vi "Condition _string_4_prod_count_month.vi"(0 "From Date":timestamp format="%<%Y-%m-%d>T", 1 "Select Stakeholder":string(combo), 5 "To Date":timestamp format="%<%Y-%m-%d>T", 7 "Shift":string(combo)="ALL", 9 "Select Station":string(combo)="ST 1", 11 "STACKHOLDER_ID":i32, 12 "Refnum out 2":T1) -> (3 "Count":i32, 4 "sum":i32[](array[numeric]), 6 "ALL IN ONE":string[][](array[string]), 8 "Table":string[][](array[string]), 10 "Elements Found out":string[](array[string]), 13 "PROD_COUNT TEST":string[](array[string]), 14 "Refnum out":T1, 15 "Array 3":string[][](array[string]))   [LabVIEW 2017]
uses:
  <vilib>/addons/database/Connection.llb/Conn ObjectReference.ctl
  <vilib>/addons/database/NI_Database_API.lvlib
panel:
  in  "Array":string[](array[string])=["1", "2", "3", "4", "5", "6"]
  out "1":string[][](array[string])
  out "6":string[][](array[string])
  out "5":string[][](array[string])
  out "4":string[][](array[string])
  out "3":string[][](array[string])
  out "2":string[][](array[string])
  out "Array 2":string[][](array[string])
  in  "String":string="Select PLAN_DATE,PRODUCTION_COUNT,STATION_ID,DATE from "
  out "error out":errorcluster
  in  "error in (no error)":errorcluster
  # "2324"
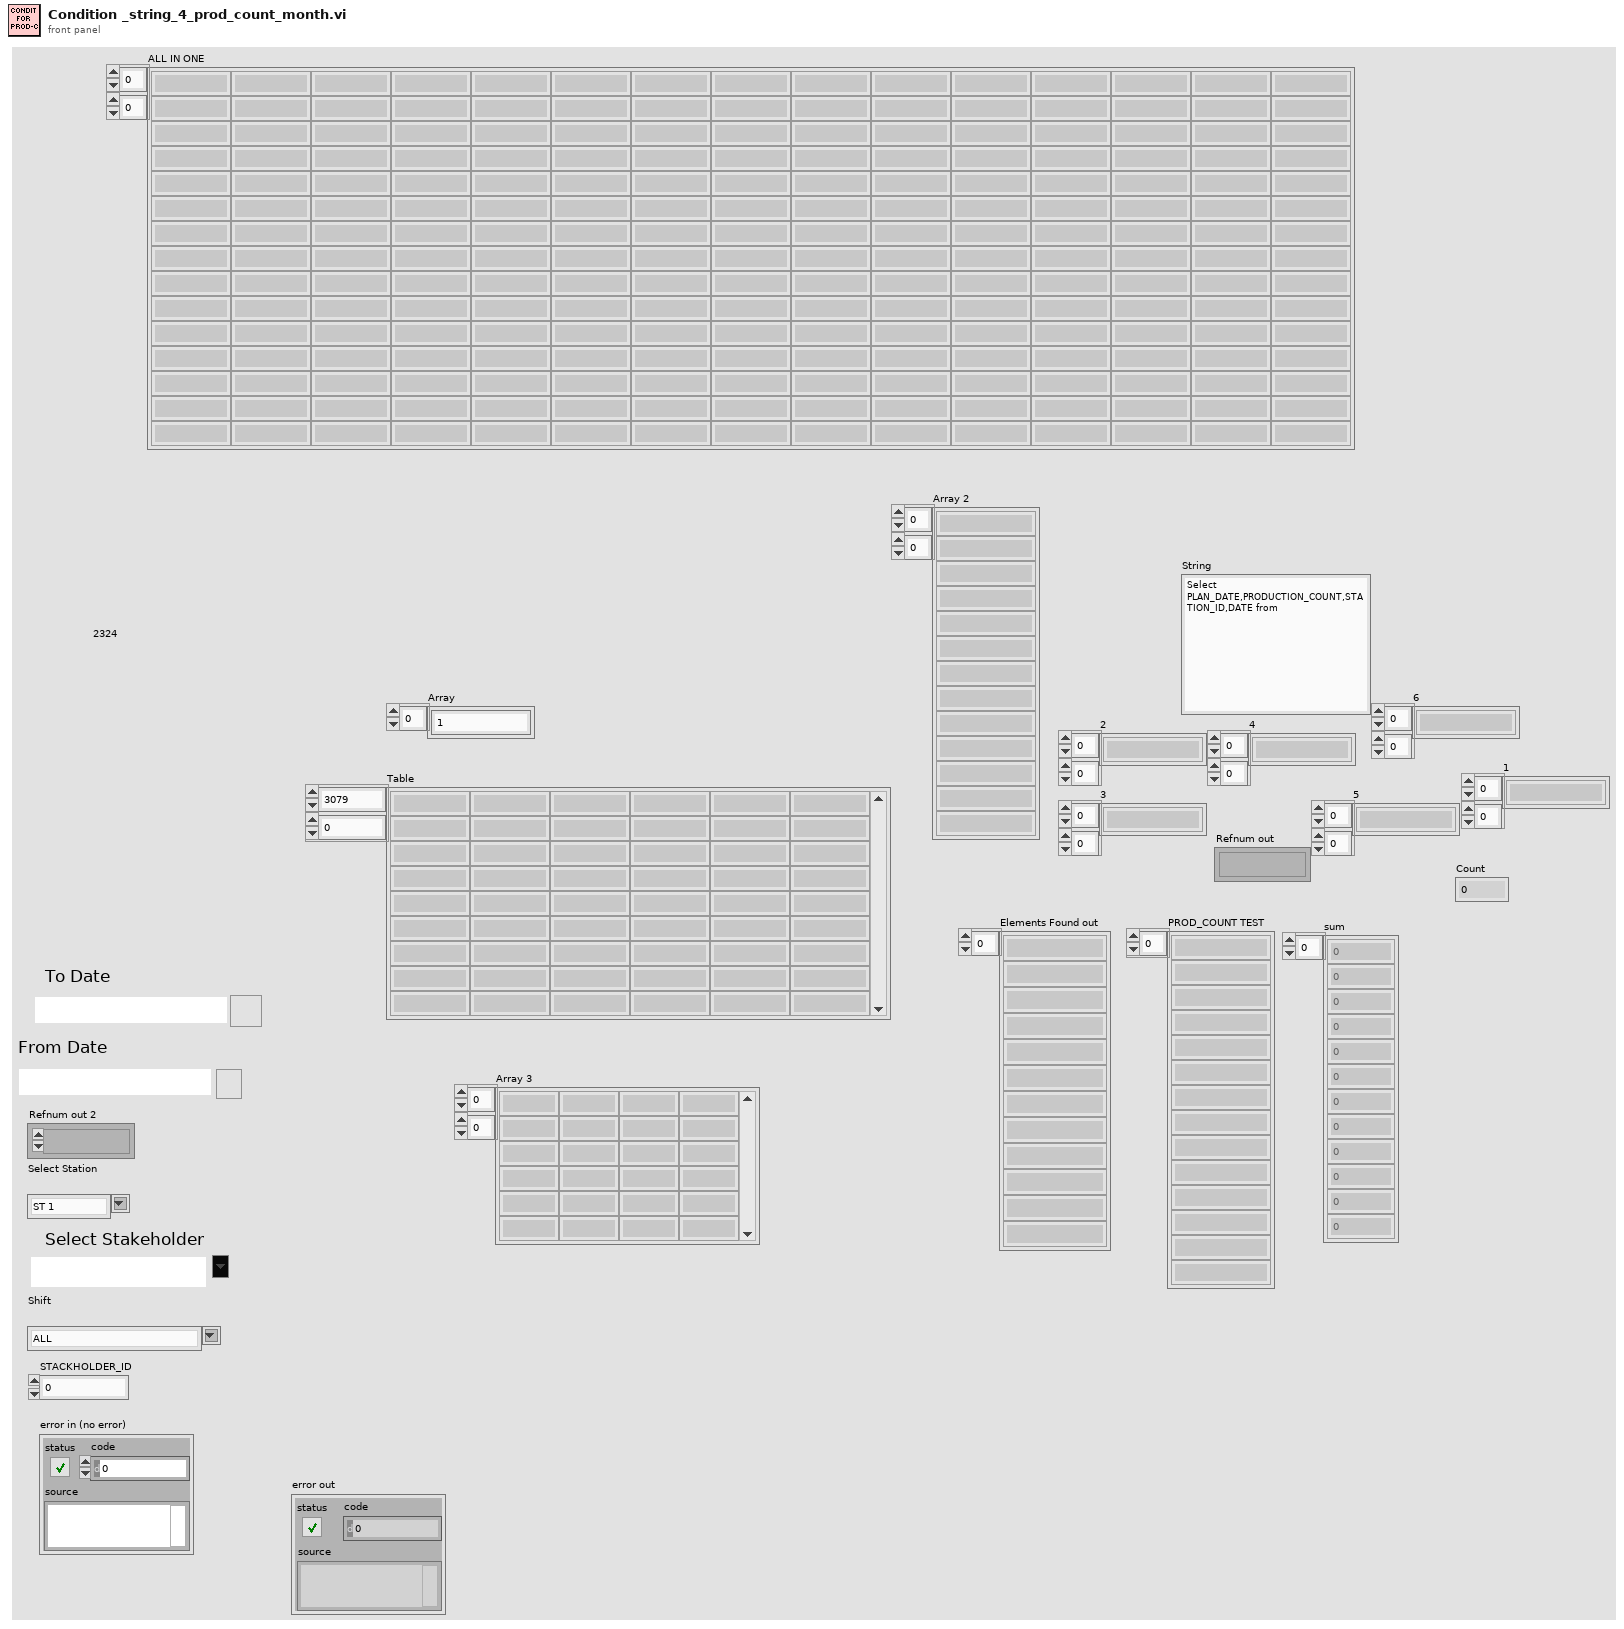
[diagram p1: front panel]
types:
  T1 = typedef "NI_Database_API.lvlib/Conn ObjectReference.ctl" = refnum<k1>
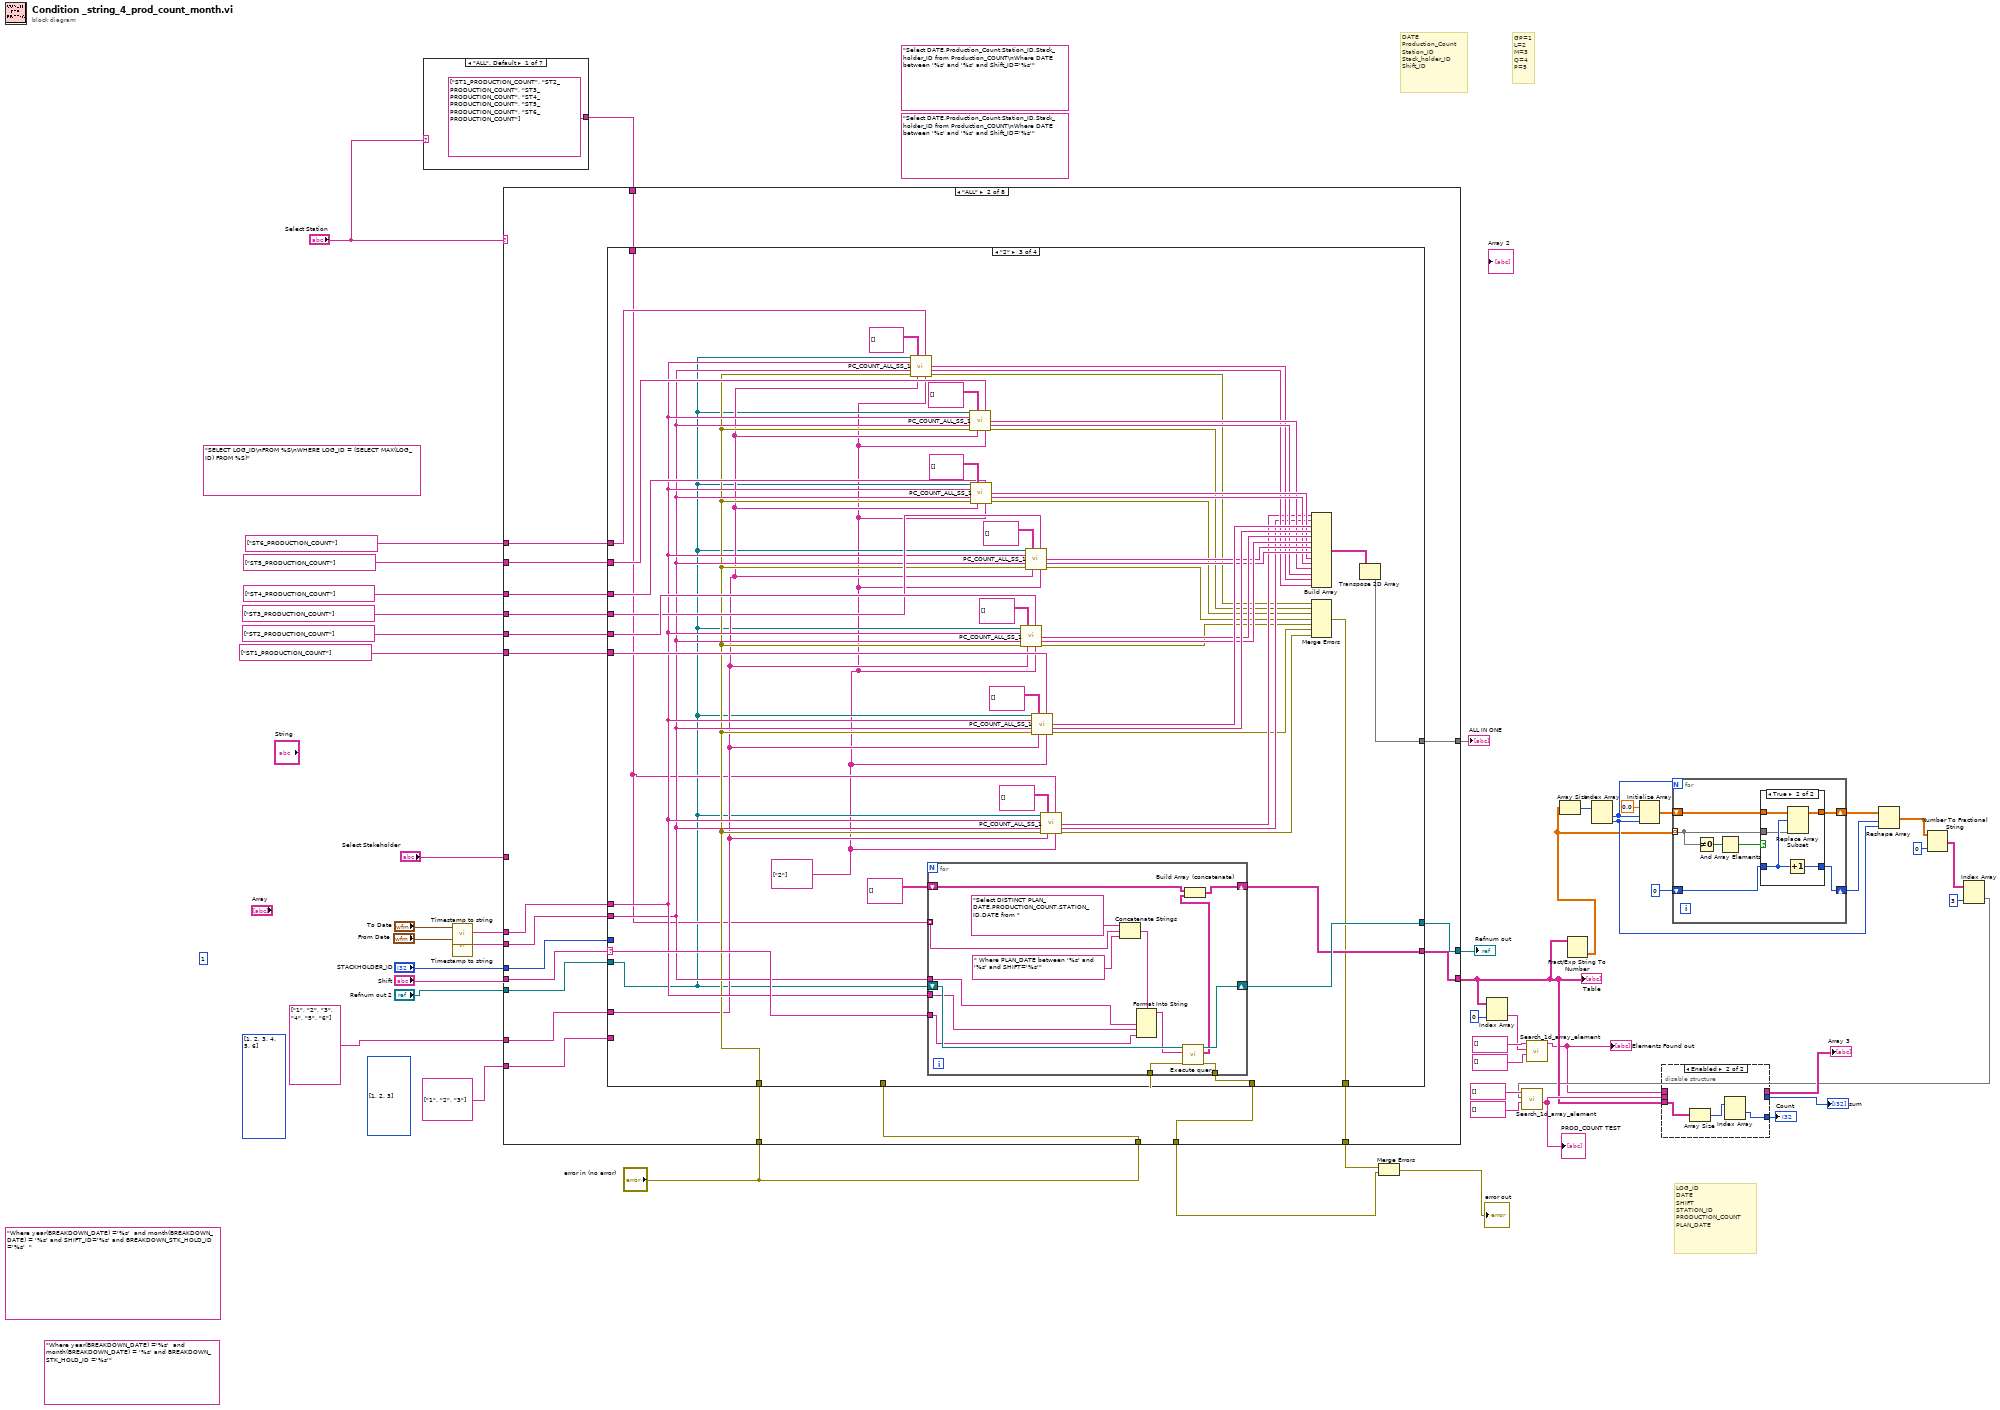
[diagram p0: block diagram]
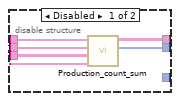
[diagram p2: hidden frame]
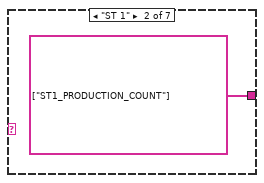
[diagram p4: hidden frame]
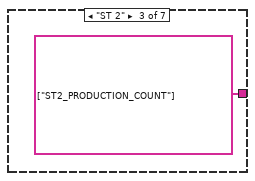
[diagram p5: hidden frame]
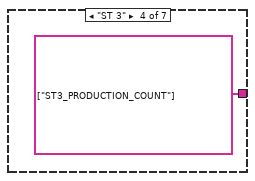
[diagram p6: hidden frame]
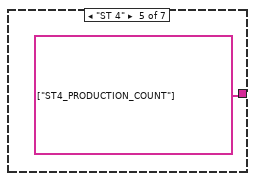
[diagram p7: hidden frame]
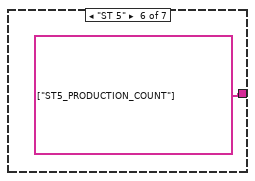
[diagram p8: hidden frame]
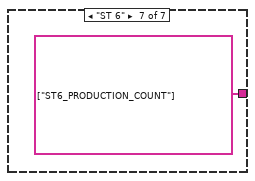
[diagram p9: hidden frame]
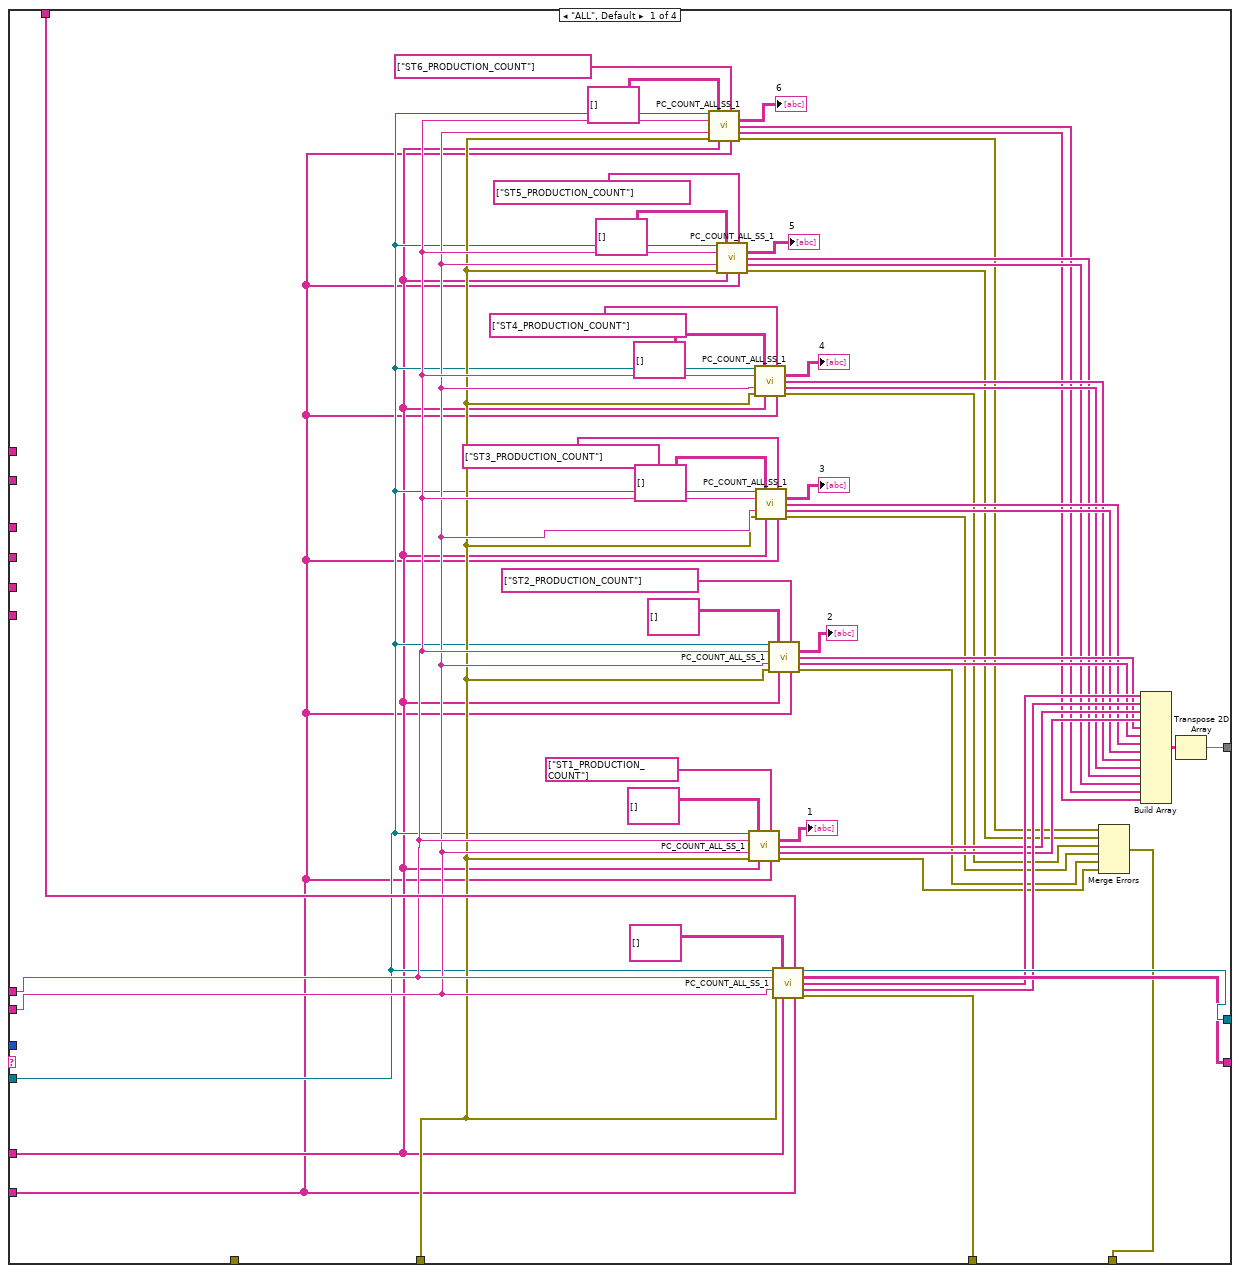
[diagram p11: hidden frame]
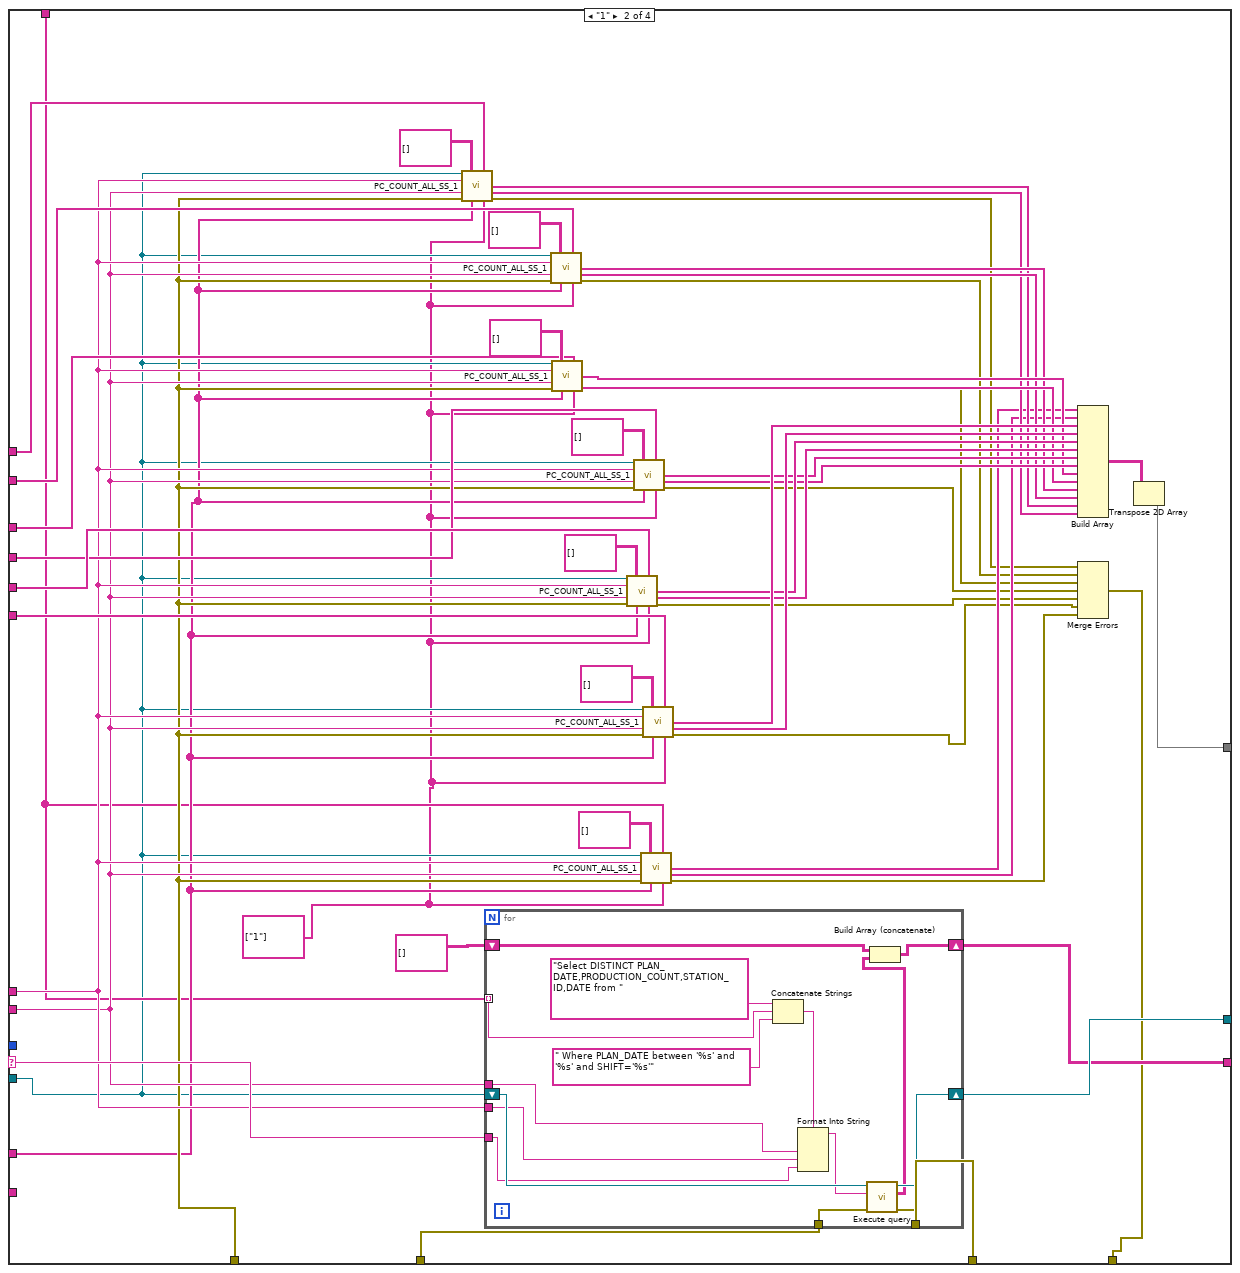
[diagram p12: hidden frame]
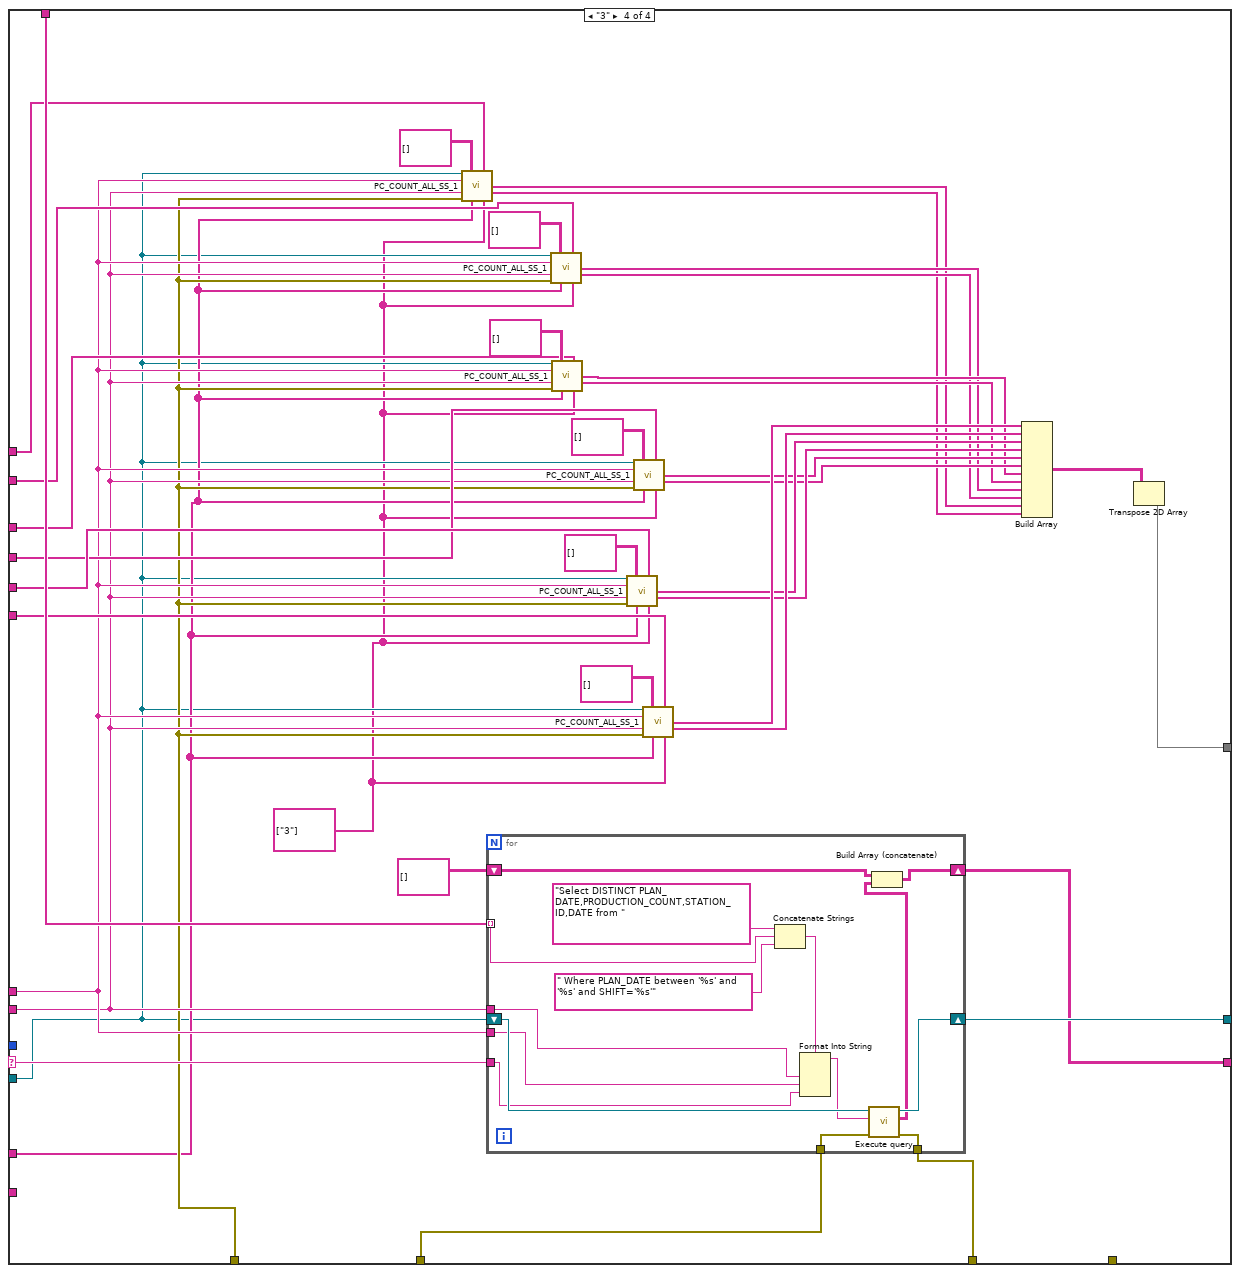
[diagram p13: hidden frame]
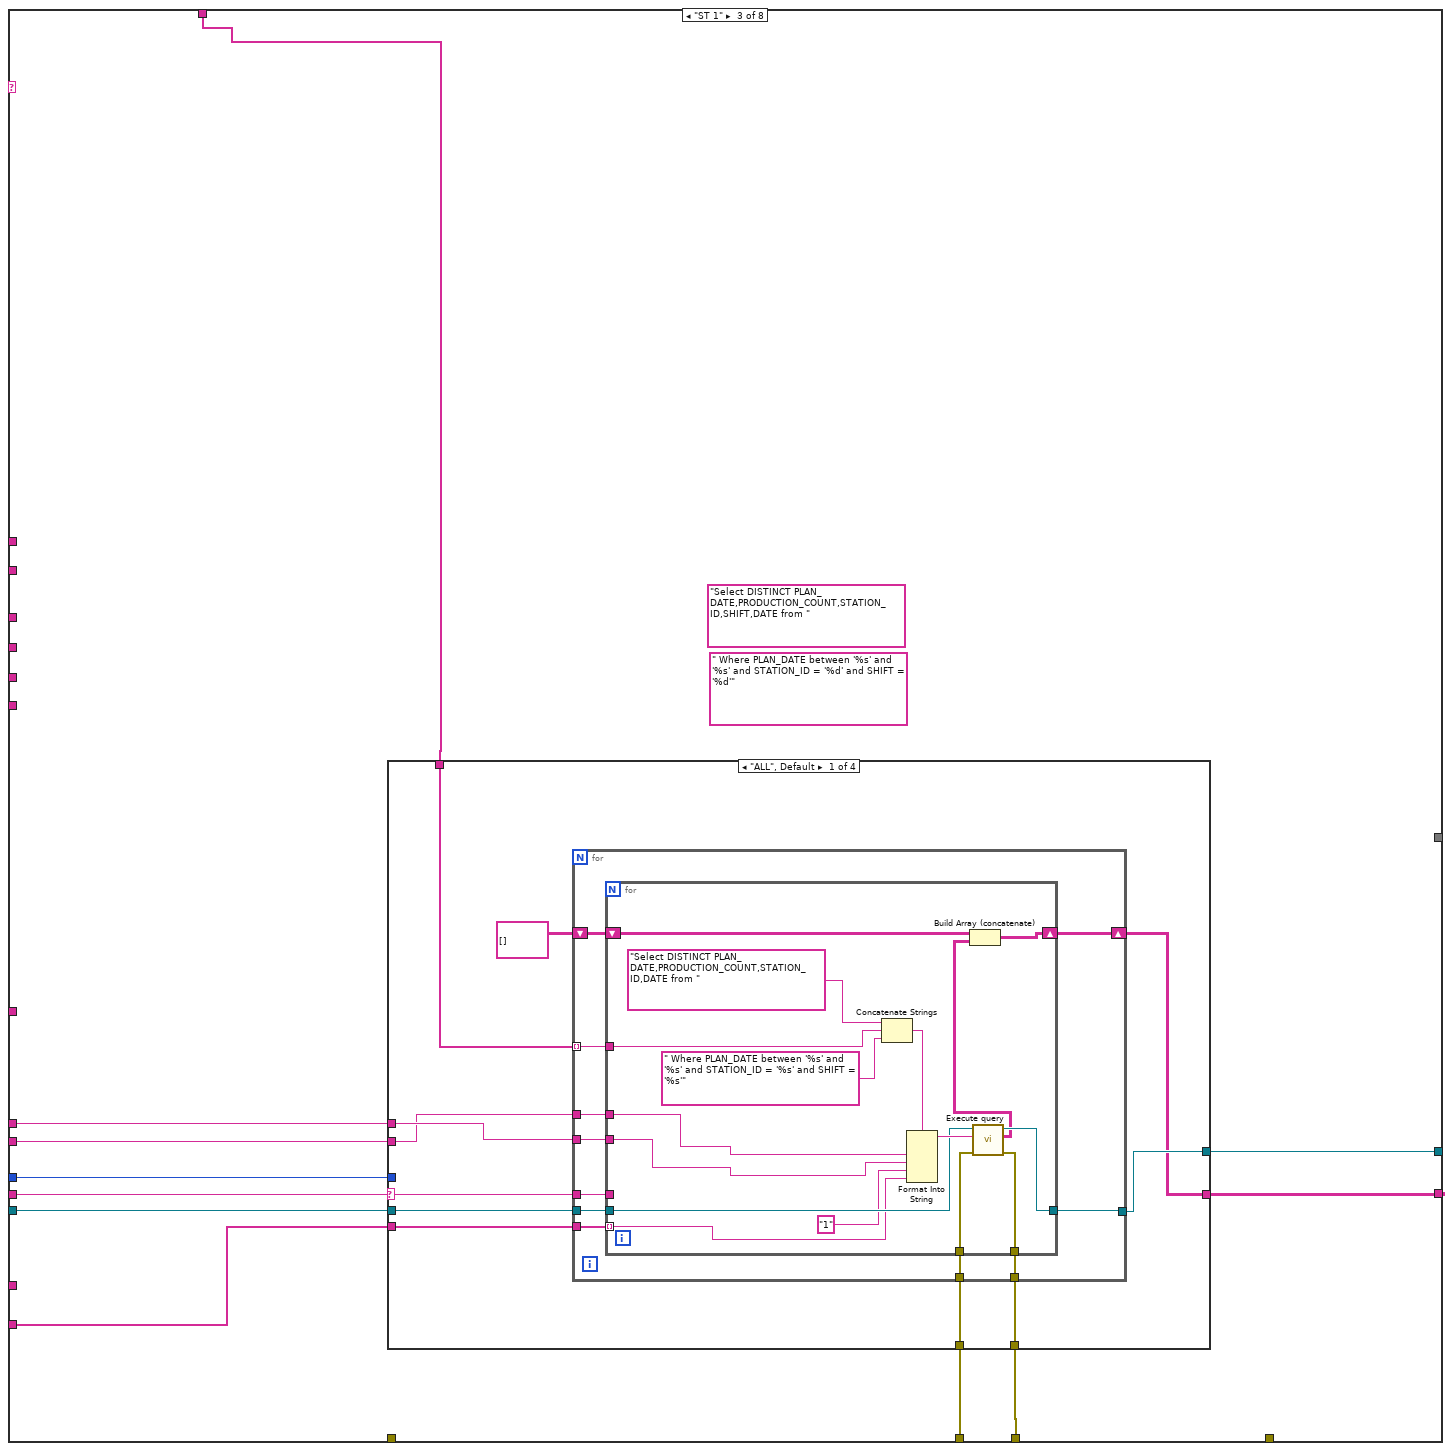
[diagram p14: hidden frame]
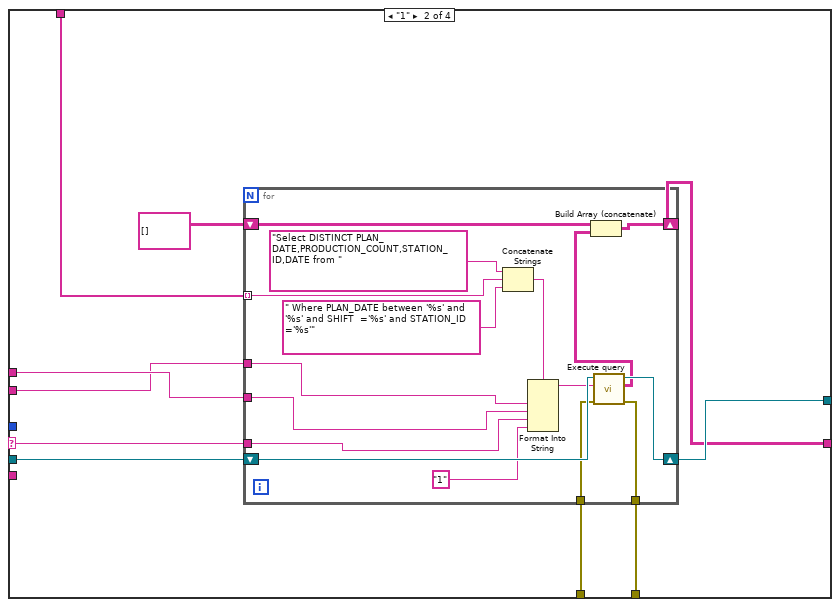
[diagram p15: hidden frame]
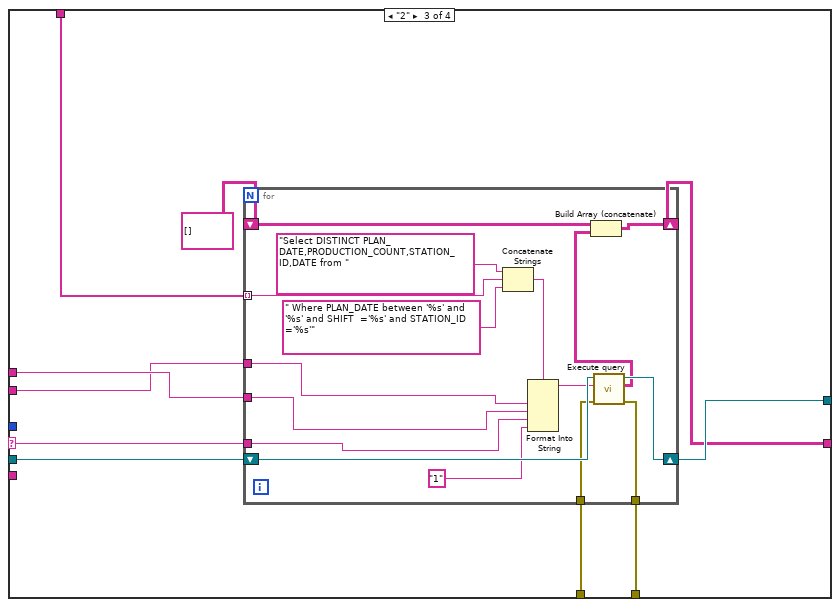
[diagram p16: hidden frame]
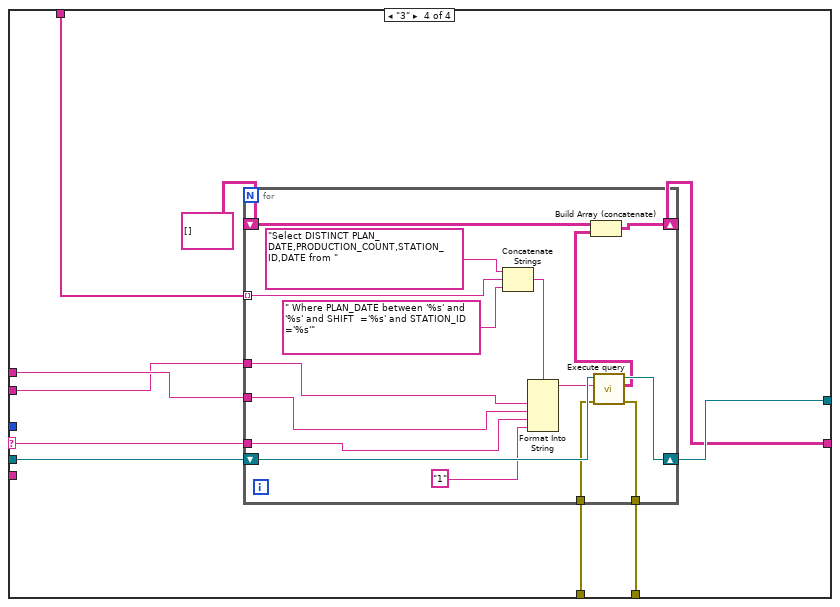
[diagram p17: hidden frame]
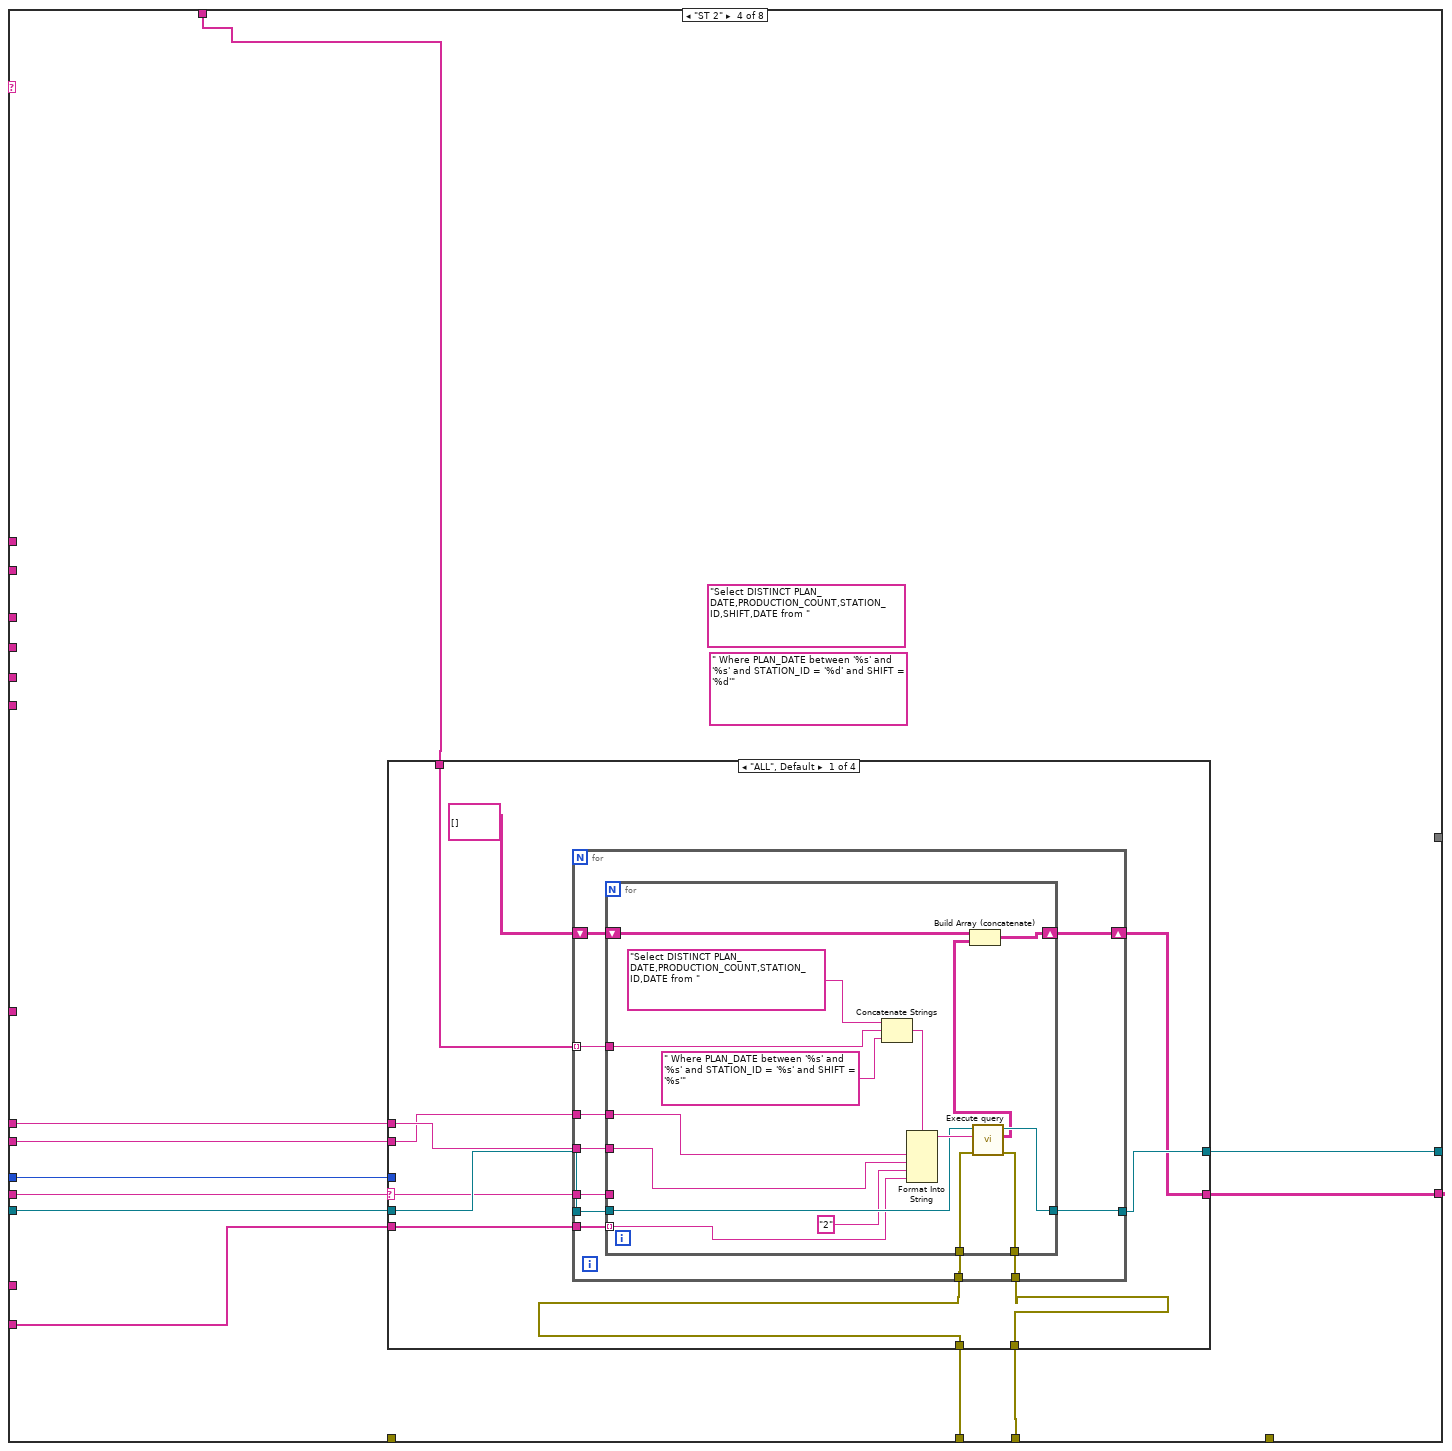
[diagram p18: hidden frame]
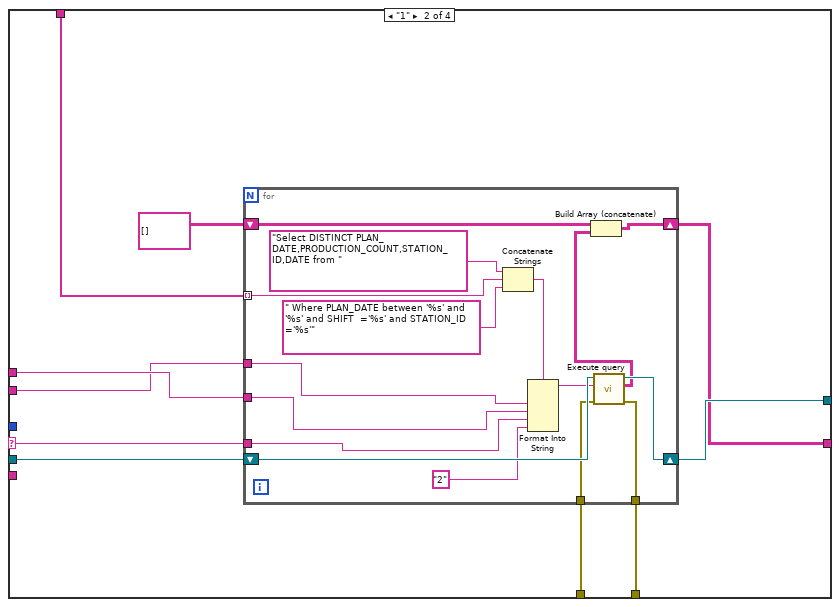
[diagram p19: hidden frame]
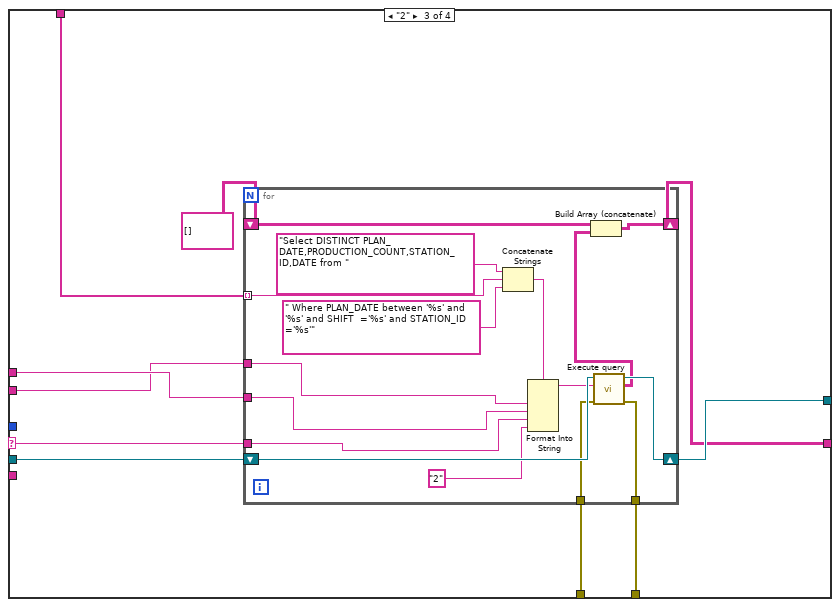
[diagram p20: hidden frame]
diagram:
  (unwired) 1
  (unwired) i32[] [1, 2, 3]
  (unwired) "SELECT LOG_ID\nFROM %S\nWHERE LOG_ID = (SELECT MAX(LOG_ID) FROM %S)" ("SQL query")
  (unwired) i32[] [1, 2, 3, 4, 5, 6]
  (unwired) "Select DATE,Production_Count,Station_ID,Stack_holder_ID from Production_COUNT\nWhere DATE between '%s' and '%s' and Shift_ID='%s'" ("string")
  (unwired) "Select DATE,Production_Count,Station_ID,Stack_holder_ID from Production_COUNT\nWhere DATE between '%s' and '%s' and Shift_ID='%s'" ("string")
  (unwired) "Where year(BREAKDOWN_DATE) ='%s'  and month(BREAKDOWN_DATE) = '%s' and BREAKDOWN_STK_HOLD_ID ='%s'" ("condition")
  (unwired) "Where year(BREAKDOWN_DATE) ='%s'  and month(BREAKDOWN_DATE) = '%s' and SHIFT_ID='%s' and BREAKDOWN_STK_HOLD_ID ='%s'  " ("condition")
  # "LOG_ID\nDATE\nSHIFT\nSTATION_ID\nPRODUCTION_COUNT\nPLAN_DATE"
  # "GP=1\nL=2\nM=3\nQ=4\nP=5"
  # "DATE\nProduction_Count\nStation_ID\nStack_holder_ID\nShift_ID"
  n1 = case shown="\"ALL\", Default" "Select Station" {
    tunnel: [string[] ["ST1_PRODUCTION_COUNT", "ST2_PRODUCTION_COUNT", "ST3_PRODUCTION_COUNT", "ST4_PRODUCTION_COUNT", "ST5_PRODUCTION_COUNT", "ST6_PRODUCTION_COUNT"] string[] ["ST1_PRODUCTION_COUNT"] string[] ["ST2_PRODUCTION_COUNT"] string[] ["ST3_PRODUCTION_COUNT"] string[] ["ST4_PRODUCTION_COUNT"] string[] ["ST5_PRODUCTION_COUNT"] string[] ["ST6_PRODUCTION_COUNT"]] -> w40
    frame "ALL", Default {
    }
    frame "ST 1" {
    }
    frame "ST 2" {
    }
    frame "ST 3" {
    }
    frame "ST 4" {
    }
    frame "ST 5" {
    }
    frame "ST 6" {
    }
  }
  n2 = call "Timestamp to string.vi"("time stamp"="To Date") -> ("Date"=w7:string)  [unwired: 8 in, 2 out]
  n3 = call "Timestamp to string.vi"("time stamp"="From Date") -> ("Date"=w5:string)  [unwired: 8 in, 2 out]
  n4 = case shown="\"ALL\"" "Select Station" {
    tunnel: "Shift" -> [_ w79 w326 w453 w580 w707 w834 w961]
    tunnel: w7 -> [_ w78 w325 w452 w579 w706 w833 w960]
    tunnel: w5 -> [_ w77 w324 w451 w578 w705 w832 w959]
    tunnel: "STACKHOLDER_ID" -> [_ w76 w323 w450 w577 w704 w831 w958]
    tunnel: [_ w75 w322 w449 w576 w703 w830 w957] -> w18
    tunnel: "Refnum out 2" -> [w58 w74 w321 w448 w575 w702 w829 w956]
    tunnel: [w58 w73 w320 w447 w574 w701 w828 w955] -> w47
    tunnel: "Select Stakeholder" -> [_ _ _ _ _ _ _ _]
    tunnel: w40 -> [_ w72 w319 w446 w573 w700 w827 w954]
    tunnel: "error in (no error)" -> [_ w71 w318 w445 w572 w699 w826 w953]
    tunnel: [_ w70 w317 w444 w571 w698 w825 w952] -> w28
    tunnel: string[] ["1", "2", "3", "4", "5", "6"] -> [_ w69 _ _ _ _ _ _]
    tunnel: string[] ["1", "2", "3"] -> [_ w68 w316 w443 w570 w697 w824 w951]
    tunnel: "error in (no error)" -> [_ w67 _ _ _ _ _ _]
    tunnel: [_ w66 _ _ _ _ _ _] -> w36
    tunnel: string[] ["ST1_PRODUCTION_COUNT"] ("Array 3") -> [_ w65 _ _ _ _ _ _]
    tunnel: string[] ["ST2_PRODUCTION_COUNT"] ("Array 3") -> [_ w64 _ _ _ _ _ _]
    tunnel: string[] ["ST3_PRODUCTION_COUNT"] ("Array 3") -> [_ w63 _ _ _ _ _ _]
    tunnel: string[] ["ST4_PRODUCTION_COUNT"] ("Array 3") -> [_ w62 _ _ _ _ _ _]
    tunnel: string[] ["ST5_PRODUCTION_COUNT"] ("Array 3") -> [_ w61 _ _ _ _ _ _]
    tunnel: string[] ["ST6_PRODUCTION_COUNT"] ("Array 3") -> [_ w60 _ _ _ _ _ _]
    tunnel: [_ w59 _ _ _ _ _ _] -> w29
    frame "False", Default {
    }
    frame "ALL" {
      n5 = case shown="\"2\"" w79 {
        selector: w79 -> [_ w180 w245 w299]
        tunnel: w78 -> [w110 w148 w213 w279]
        tunnel: w77 -> [w109 w147 w212 w278]
        tunnel: w76 -> [_ _ _ _]
        tunnel: [w127 w178 w243 w296] -> w75
        tunnel: w74 -> [w96 w141 w206 w275]
        tunnel: [w131 w181 w246 w300] -> w73
        tunnel: w72 -> [w130 w144 w209 w298]
        tunnel: w71 -> [w108 w177 w242 w295]
        tunnel: [w128 w176 w241 w294] -> w70
        tunnel: w69 -> [w94 w145 w210 w276]
        tunnel: w68 -> [w93 _ _ _]
        tunnel: w67 -> [_ w146 w211 w277]
        tunnel: [w95 w150 w215 w263] -> w66
        tunnel: w65 -> [_ w175 w240 w293]
        tunnel: w64 -> [_ w166 w231 w284]
        tunnel: w63 -> [_ w165 w230 w283]
        tunnel: w62 -> [_ w164 w229 w282]
        tunnel: w61 -> [_ w163 w228 w281]
        tunnel: w60 -> [_ w162 w227 w280]
        tunnel: [w86 w133 w198 _] -> w59
        frame "ALL", Default {
          n6 = call "PC_COUNT_ALL_SS_1.vi"("Refnum in"=w96, "data in"=string[][] [] ("data"), "Array 3"=string[] ["ST6_PRODUCTION_COUNT"], "To Date"=w110, "From Date"=w109, "error in (no error)"=w108, "Station"=w94, "Shift"=w93) -> ("data out"=→"6":string[][], "DATE"=w99:string[], "COUNT"=w98:string[], "error out"=w92:errorcluster)  [unwired: 3 in, 1 out]
          n7 = call "PC_COUNT_ALL_SS_1.vi"("Refnum in"=w96, "data in"=string[][] [] ("data"), "Array 3"=string[] ["ST5_PRODUCTION_COUNT"], "To Date"=w110, "From Date"=w109, "error in (no error)"=w108, "Station"=w94, "Shift"=w93) -> ("data out"=→"5":string[][], "DATE"=w101:string[], "COUNT"=w100:string[], "error out"=w91:errorcluster)  [unwired: 3 in, 1 out]
          n8 = call "PC_COUNT_ALL_SS_1.vi"("Refnum in"=w96, "data in"=string[][] [] ("data"), "Array 3"=string[] ["ST1_PRODUCTION_COUNT"], "To Date"=w110, "From Date"=w109, "error in (no error)"=w108, "Station"=w94, "Shift"=w93) -> ("data out"=→"1":string[][], "DATE"=w122:string[], "COUNT"=w121:string[], "error out"=w87:errorcluster)  [unwired: 3 in, 1 out]
          n9 = call "PC_COUNT_ALL_SS_1.vi"("Refnum in"=w96, "data in"=string[][] [] ("data"), "Array 3"=string[] ["ST4_PRODUCTION_COUNT"], "To Date"=w110, "From Date"=w109, "error in (no error)"=w108, "Station"=w94, "Shift"=w93) -> ("data out"=→"4":string[][], "DATE"=w103:string[], "COUNT"=w102:string[], "error out"=w90:errorcluster)  [unwired: 3 in, 1 out]
          n10 = call "PC_COUNT_ALL_SS_1.vi"("Refnum in"=w96, "data in"=string[][] [] ("data"), "Array 3"=string[] ["ST3_PRODUCTION_COUNT"], "To Date"=w110, "From Date"=w109, "error in (no error)"=w108, "Station"=w94, "Shift"=w93) -> ("data out"=→"3":string[][], "DATE"=w105:string[], "COUNT"=w104:string[], "error out"=w89:errorcluster)  [unwired: 3 in, 1 out]
          n11 = call "PC_COUNT_ALL_SS_1.vi"("Refnum in"=w96, "data in"=string[][] [] ("data"), "Array 3"=string[] ["ST2_PRODUCTION_COUNT"], "To Date"=w110, "From Date"=w109, "error in (no error)"=w108, "Station"=w94, "Shift"=w93) -> ("data out"=→"2":string[][], "DATE"=w118:string[], "COUNT"=w117:string[], "error out"=w88:errorcluster)  [unwired: 3 in, 1 out]
          n12 = call "PC_COUNT_ALL_SS_1.vi"("Refnum in"=w96, "data in"=string[][] [] ("data"), "Array 3"=w130, "To Date"=w110, "From Date"=w109, "error in (no error)"=w108, "Station"=w94, "Shift"=w93) -> ("Refnum out"=w131:T1, "data out"=w127:string[][], "DATE"=w124:string[], "COUNT"=w123:string[], "error out"=w128:errorcluster)  [unwired: 3 in]
          n13 = Merge Errors(w92, w91, w90, w89, w88, w87) -> (w86:errorcluster)
          n14 = Build Array(w124, w123, w122, w121, w118, w117, w105, w104, w103, w102, w101, w100, w99, w98) -> (w97:string[][])
          n15 = Transpose 2D Array(2D array=w97) -> (transposed array=w95:string[][])
        }
        frame "1" {
          w132 = string[] ["1"]
          n16 = call "PC_COUNT_ALL_SS_1.vi"("Refnum in"=w141, "data in"=string[][] [], "Array 3"=w162, "To Date"=w148, "From Date"=w147, "error in (no error)"=w146, "Station"=w145, "Shift"=w132) -> ("DATE"=w153:string[], "COUNT"=w152:string[], "error out"=w140:errorcluster)  [unwired: 3 in, 2 out]
          n17 = for {
            tunnel: w148 -> [w182]
            tunnel: w147 -> [w183]
            tunnel: w180 -> [w193]
            shift-right: [w194] -> w181
            shift-left: w141 -> [w196]
            tunnel: w144 -> [w191] mode=indexing
            shift-right: [w187] -> w178
            shift-left: string[][] [] ("data") -> [w188]
            tunnel: w177 -> [w185]
            tunnel: [w184] -> w176
            n18 = Concatenate Strings("Select DISTINCT PLAN_DATE,PRODUCTION_COUNT,STATION_ID,DATE from ", w191, " Where PLAN_DATE between '%s' and '%s' and SHIFT='%s'") -> (w192:string)
            n19 = Format Into String(format string=w192, w183, w182, w193) -> (resulting string=w195:string)  [unwired: 2 in, 1 out]
            n20 = call "Execute query.vi"("error in (no error)"=w185, "String"=w195, "connection reference"=w196) -> ("error out"=w184:errorcluster, "Table"=w186:string[][], "connection reference 2"=w194:T1)  [unwired: 3 in, 3 out]
            n21 = Build Array (concatenate)(w188, w186) -> (w187:string[][])
          }
          n22 = call "PC_COUNT_ALL_SS_1.vi"("Refnum in"=w141, "data in"=string[][] [], "Array 3"=w163, "To Date"=w148, "From Date"=w147, "error in (no error)"=w146, "Station"=w145, "Shift"=w132) -> ("DATE"=w155:string[], "COUNT"=w154:string[], "error out"=w139:errorcluster)  [unwired: 3 in, 2 out]
          n23 = call "PC_COUNT_ALL_SS_1.vi"("Refnum in"=w141, "data in"=string[][] [], "Array 3"=w164, "To Date"=w148, "From Date"=w147, "error in (no error)"=w146, "Station"=w145, "Shift"=w132) -> ("DATE"=w157:string[], "COUNT"=w156:string[], "error out"=w138:errorcluster)  [unwired: 3 in, 2 out]
          n24 = call "PC_COUNT_ALL_SS_1.vi"("Refnum in"=w141, "data in"=string[][] [], "Array 3"=w166, "To Date"=w148, "From Date"=w147, "error in (no error)"=w146, "Station"=w145, "Shift"=w132) -> ("DATE"=w161:string[], "COUNT"=w160:string[], "error out"=w136:errorcluster)  [unwired: 3 in, 2 out]
          n25 = call "PC_COUNT_ALL_SS_1.vi"("Refnum in"=w141, "data in"=string[][] [], "Array 3"=w165, "To Date"=w148, "From Date"=w147, "error in (no error)"=w146, "Station"=w145, "Shift"=w132) -> ("DATE"=w159:string[], "COUNT"=w158:string[], "error out"=w137:errorcluster)  [unwired: 3 in, 2 out]
          n26 = call "PC_COUNT_ALL_SS_1.vi"("Refnum in"=w141, "data in"=string[][] [], "Array 3"=w144, "To Date"=w148, "From Date"=w147, "error in (no error)"=w146, "Station"=w145, "Shift"=w132) -> ("DATE"=w143:string[], "COUNT"=w142:string[], "error out"=w134:errorcluster)  [unwired: 3 in, 2 out]
          n27 = call "PC_COUNT_ALL_SS_1.vi"("Refnum in"=w141, "data in"=string[][] [], "Array 3"=w175, "To Date"=w148, "From Date"=w147, "error in (no error)"=w146, "Station"=w145, "Shift"=w132) -> ("DATE"=w173:string[], "COUNT"=w172:string[], "error out"=w135:errorcluster)  [unwired: 3 in, 2 out]
          n28 = Build Array(w143, w142, w173, w172, w161, w160, w159, w158, w157, w156, w155, w154, w153, w152) -> (w151:string[][])
          n29 = Merge Errors(w140, w139, w138, w137, w136, w135, w134) -> (w133:errorcluster)
          n30 = Transpose 2D Array(2D array=w151) -> (transposed array=w150:string[][])
        }
        frame "2" {
          w197 = string[] ["2"]
          n31 = call "PC_COUNT_ALL_SS_1.vi"("Refnum in"=w206, "data in"=string[][] [], "Array 3"=w227, "To Date"=w213, "From Date"=w212, "error in (no error)"=w211, "Station"=w210, "Shift"=w197) -> ("DATE"=w218:string[], "COUNT"=w217:string[], "error out"=w205:errorcluster)  [unwired: 3 in, 2 out]
          n32 = for {
            tunnel: w213 -> [w247]
            tunnel: w212 -> [w248]
            tunnel: w245 -> [w258]
            shift-right: [w259] -> w246
            shift-left: w206 -> [w261]
            tunnel: w209 -> [w256] mode=indexing
            shift-right: [w252] -> w243
            shift-left: string[][] [] ("data") -> [w253]
            tunnel: w242 -> [w250]
            tunnel: [w249] -> w241
            n33 = Concatenate Strings("Select DISTINCT PLAN_DATE,PRODUCTION_COUNT,STATION_ID,DATE from ", w256, " Where PLAN_DATE between '%s' and '%s' and SHIFT='%s'") -> (w257:string)
            n34 = Format Into String(format string=w257, w248, w247, w258) -> (resulting string=w260:string)  [unwired: 2 in, 1 out]
            n35 = call "Execute query.vi"("error in (no error)"=w250, "String"=w260, "connection reference"=w261) -> ("error out"=w249:errorcluster, "Table"=w251:string[][], "connection reference 2"=w259:T1)  [unwired: 3 in, 3 out]
            n36 = Build Array (concatenate)(w253, w251) -> (w252:string[][])
          }
          n37 = call "PC_COUNT_ALL_SS_1.vi"("Refnum in"=w206, "data in"=string[][] [], "Array 3"=w228, "To Date"=w213, "From Date"=w212, "error in (no error)"=w211, "Station"=w210, "Shift"=w197) -> ("DATE"=w220:string[], "COUNT"=w219:string[], "error out"=w204:errorcluster)  [unwired: 3 in, 2 out]
          n38 = call "PC_COUNT_ALL_SS_1.vi"("Refnum in"=w206, "data in"=string[][] [], "Array 3"=w229, "To Date"=w213, "From Date"=w212, "error in (no error)"=w211, "Station"=w210, "Shift"=w197) -> ("DATE"=w222:string[], "COUNT"=w221:string[], "error out"=w203:errorcluster)  [unwired: 3 in, 2 out]
          n39 = call "PC_COUNT_ALL_SS_1.vi"("Refnum in"=w206, "data in"=string[][] [], "Array 3"=w231, "To Date"=w213, "From Date"=w212, "error in (no error)"=w211, "Station"=w210, "Shift"=w197) -> ("DATE"=w226:string[], "COUNT"=w225:string[], "error out"=w201:errorcluster)  [unwired: 3 in, 2 out]
          n40 = call "PC_COUNT_ALL_SS_1.vi"("Refnum in"=w206, "data in"=string[][] [], "Array 3"=w230, "To Date"=w213, "From Date"=w212, "error in (no error)"=w211, "Station"=w210, "Shift"=w197) -> ("DATE"=w224:string[], "COUNT"=w223:string[], "error out"=w202:errorcluster)  [unwired: 3 in, 2 out]
          n41 = call "PC_COUNT_ALL_SS_1.vi"("Refnum in"=w206, "data in"=string[][] [], "Array 3"=w240, "To Date"=w213, "From Date"=w212, "error in (no error)"=w211, "Station"=w210, "Shift"=w197) -> ("DATE"=w238:string[], "COUNT"=w237:string[], "error out"=w200:errorcluster)  [unwired: 3 in, 2 out]
          n42 = call "PC_COUNT_ALL_SS_1.vi"("Refnum in"=w206, "data in"=string[][] [], "Array 3"=w209, "To Date"=w213, "From Date"=w212, "error in (no error)"=w211, "Station"=w210, "Shift"=w197) -> ("DATE"=w208:string[], "COUNT"=w207:string[], "error out"=w199:errorcluster)  [unwired: 3 in, 2 out]
          n43 = Build Array(w208, w207, w238, w237, w226, w225, w224, w223, w222, w221, w220, w219, w218, w217) -> (w216:string[][])
          n44 = Merge Errors(w205, w204, w203, w202, w201, w200, w199) -> (w198:errorcluster)
          n45 = Transpose 2D Array(2D array=w216) -> (transposed array=w215:string[][])
        }
        frame "3" {
          w262 = string[] ["3"]
          n46 = call "PC_COUNT_ALL_SS_1.vi"("Refnum in"=w275, "data in"=string[][] [], "Array 3"=w280, "To Date"=w279, "From Date"=w278, "error in (no error)"=w277, "Station"=w276, "Shift"=w262) -> ("DATE"=w266:string[], "COUNT"=w265:string[])  [unwired: 3 in, 3 out]
          n47 = for {
            tunnel: w279 -> [w301]
            tunnel: w278 -> [w302]
            tunnel: w299 -> [w312]
            shift-right: [w313] -> w300
            shift-left: w275 -> [w315]
            tunnel: w298 -> [w310] mode=indexing
            shift-right: [w306] -> w296
            shift-left: string[][] [] ("data") -> [w307]
            tunnel: w295 -> [w304]
            tunnel: [w303] -> w294
            n48 = Concatenate Strings("Select DISTINCT PLAN_DATE,PRODUCTION_COUNT,STATION_ID,DATE from ", w310, " Where PLAN_DATE between '%s' and '%s' and SHIFT='%s'") -> (w311:string)
            n49 = Format Into String(format string=w311, w302, w301, w312) -> (resulting string=w314:string)  [unwired: 2 in, 1 out]
            n50 = call "Execute query.vi"("error in (no error)"=w304, "String"=w314, "connection reference"=w315) -> ("error out"=w303:errorcluster, "Table"=w305:string[][], "connection reference 2"=w313:T1)  [unwired: 3 in, 3 out]
            n51 = Build Array (concatenate)(w307, w305) -> (w306:string[][])
          }
          n52 = call "PC_COUNT_ALL_SS_1.vi"("Refnum in"=w275, "data in"=string[][] [], "Array 3"=w281, "To Date"=w279, "From Date"=w278, "error in (no error)"=w277, "Station"=w276, "Shift"=w262) -> ("DATE"=w268:string[], "COUNT"=w267:string[])  [unwired: 3 in, 3 out]
          n53 = call "PC_COUNT_ALL_SS_1.vi"("Refnum in"=w275, "data in"=string[][] [], "Array 3"=w282, "To Date"=w279, "From Date"=w278, "error in (no error)"=w277, "Station"=w276, "Shift"=w262) -> ("DATE"=w270:string[], "COUNT"=w269:string[])  [unwired: 3 in, 3 out]
          n54 = call "PC_COUNT_ALL_SS_1.vi"("Refnum in"=w275, "data in"=string[][] [], "Array 3"=w284, "To Date"=w279, "From Date"=w278, "error in (no error)"=w277, "Station"=w276, "Shift"=w262) -> ("DATE"=w274:string[], "COUNT"=w273:string[])  [unwired: 3 in, 3 out]
          n55 = call "PC_COUNT_ALL_SS_1.vi"("Refnum in"=w275, "data in"=string[][] [], "Array 3"=w283, "To Date"=w279, "From Date"=w278, "error in (no error)"=w277, "Station"=w276, "Shift"=w262) -> ("DATE"=w272:string[], "COUNT"=w271:string[])  [unwired: 3 in, 3 out]
          n56 = call "PC_COUNT_ALL_SS_1.vi"("Refnum in"=w275, "data in"=string[][] [], "Array 3"=w293, "To Date"=w279, "From Date"=w278, "error in (no error)"=w277, "Station"=w276, "Shift"=w262) -> ("DATE"=w291:string[], "COUNT"=w290:string[])  [unwired: 3 in, 3 out]
          n57 = Build Array(w291, w290, w274, w273, w272, w271, w270, w269, w268, w267, w266, w265) -> (w264:string[][])
          n58 = Transpose 2D Array(2D array=w264) -> (transposed array=w263:string[][])
        }
      }
    }
    frame "ST 1" {
      (unwired) "Select DISTINCT PLAN_DATE,PRODUCTION_COUNT,STATION_ID,SHIFT,DATE from "
      (unwired) " Where PLAN_DATE between '%s' and '%s' and STATION_ID = '%d' and SHIFT = '%d'"
      n59 = case shown="\"ALL\", Default" w326 {
        selector: w326 -> [w333 w370 w396 w422]
        tunnel: w325 -> [w337 w374 w400 w426]
        tunnel: w324 -> [w336 w373 w399 w425]
        tunnel: w323 -> [_ _ _ _]
        tunnel: [w328 w367 w393 w419] -> w322
        tunnel: w321 -> [w335 w372 w398 w424]
        tunnel: [w334 w371 w397 w423] -> w320
        tunnel: w319 -> [w332 w369 w395 w421]
        tunnel: w318 -> [w330 w365 w392 w418]
        tunnel: [w329 w366 w391 w417] -> w317
        tunnel: w316 -> [w327 _ _ _]
        frame "ALL", Default {
          n60 = for {
            tunnel: w337 -> [w348]
            tunnel: w336 -> [w347]
            tunnel: w333 -> [w344]
            tunnel: w332 -> [w343] mode=indexing
            tunnel: w330 -> [w341]
            tunnel: [w340] -> w329
            tunnel: w335 -> [w346]
            tunnel: [w345] -> w334
            shift-right: [w339] -> w328
            shift-left: string[][] [] ("data") -> [w342]
            tunnel: w327 -> [w338]
            n61 = for {
              tunnel: w348 -> [w349]
              tunnel: w347 -> [w350]
              tunnel: w344 -> [_]
              tunnel: w343 -> [w362]
              shift-right: [w352] -> w339
              shift-left: w342 -> [w359]
              tunnel: w341 -> [w355]
              tunnel: [w354] -> w340
              tunnel: w346 -> [w357]
              tunnel: [w363] -> w345
              tunnel: w338 -> [w351] mode=indexing
              n62 = Concatenate Strings("Select DISTINCT PLAN_DATE,PRODUCTION_COUNT,STATION_ID,DATE from ", w362, " Where PLAN_DATE between '%s' and '%s' and STATION_ID = '%s' and SHIFT = '%s'") -> (w360:string)
              n63 = Format Into String(format string=w360, w350, w349, "1", w351) -> (resulting string=w364:string)  [unwired: 2 in, 1 out]
              n64 = call "Execute query.vi"("error in (no error)"=w355, "String"=w364, "connection reference"=w357) -> ("error out"=w354:errorcluster, "Table"=w358:string[][], "connection reference 2"=w363:T1)  [unwired: 3 in, 3 out]
              n65 = Build Array (concatenate)(w359, w358) -> (w352:string[][])
            }
          }
        }
        frame "1" {
          n66 = for {
            tunnel: w374 -> [w375]
            tunnel: w373 -> [w376]
            tunnel: w370 -> [w387]
            tunnel: w369 -> [w386] mode=indexing
            shift-right: [w388] -> w371
            shift-left: w372 -> [w390]
            shift-right: [w381] -> w367
            shift-left: string[][] [] ("data") -> [w383]
            tunnel: [w378] -> w366
            tunnel: w365 -> [w377]
            n67 = Concatenate Strings("Select DISTINCT PLAN_DATE,PRODUCTION_COUNT,STATION_ID,DATE from ", w386, " Where PLAN_DATE between '%s' and '%s' and SHIFT  ='%s' and STATION_ID ='%s'") -> (w384:string)
            n68 = Format Into String(format string=w384, w376, w375, w387, "1") -> (resulting string=w389:string)  [unwired: 2 in, 1 out]
            n69 = call "Execute query.vi"("error in (no error)"=w377, "String"=w389, "connection reference"=w390) -> ("error out"=w378:errorcluster, "Table"=w382:string[][], "connection reference 2"=w388:T1)  [unwired: 3 in, 3 out]
            n70 = Build Array (concatenate)(w383, w382) -> (w381:string[][])
          }
        }
        frame "2" {
          n71 = for {
            tunnel: w400 -> [w401]
            tunnel: w399 -> [w402]
            tunnel: w396 -> [w413]
            tunnel: w395 -> [w412] mode=indexing
            shift-right: [w414] -> w397
            shift-left: w398 -> [w416]
            shift-right: [w407] -> w393
            shift-left: string[][] [] ("data") -> [w409]
            tunnel: w392 -> [w404]
            tunnel: [w403] -> w391
            n72 = Concatenate Strings("Select DISTINCT PLAN_DATE,PRODUCTION_COUNT,STATION_ID,DATE from ", w412, " Where PLAN_DATE between '%s' and '%s' and SHIFT  ='%s' and STATION_ID ='%s'") -> (w410:string)
            n73 = Format Into String(format string=w410, w402, w401, w413, "1") -> (resulting string=w415:string)  [unwired: 2 in, 1 out]
            n74 = call "Execute query.vi"("error in (no error)"=w404, "String"=w415, "connection reference"=w416) -> ("error out"=w403:errorcluster, "Table"=w408:string[][], "connection reference 2"=w414:T1)  [unwired: 3 in, 3 out]
            n75 = Build Array (concatenate)(w409, w408) -> (w407:string[][])
          }
        }
        frame "3" {
          n76 = for {
            tunnel: w426 -> [w427]
            tunnel: w425 -> [w428]
            tunnel: w422 -> [w439]
            tunnel: w421 -> [w438] mode=indexing
            shift-right: [w440] -> w423
            shift-left: w424 -> [w442]
            shift-right: [w433] -> w419
            shift-left: string[][] [] ("data") -> [w435]
            tunnel: w418 -> [w430]
            tunnel: [w429] -> w417
            n77 = Concatenate Strings("Select DISTINCT PLAN_DATE,PRODUCTION_COUNT,STATION_ID,DATE from ", w438, " Where PLAN_DATE between '%s' and '%s' and SHIFT  ='%s' and STATION_ID ='%s'") -> (w436:string)
            n78 = Format Into String(format string=w436, w428, w427, w439, "1") -> (resulting string=w441:string)  [unwired: 2 in, 1 out]
            n79 = call "Execute query.vi"("error in (no error)"=w430, "String"=w441, "connection reference"=w442) -> ("error out"=w429:errorcluster, "Table"=w434:string[][], "connection reference 2"=w440:T1)  [unwired: 3 in, 3 out]
            n80 = Build Array (concatenate)(w435, w434) -> (w433:string[][])
          }
        }
      }
    }
    frame "ST 2" {
      (unwired) "Select DISTINCT PLAN_DATE,PRODUCTION_COUNT,STATION_ID,SHIFT,DATE from "
      (unwired) " Where PLAN_DATE between '%s' and '%s' and STATION_ID = '%d' and SHIFT = '%d'"
      n81 = case shown="\"ALL\", Default" w453 {
        selector: w453 -> [w460 w497 w523 w549]
        tunnel: w452 -> [w464 w501 w527 w553]
        tunnel: w451 -> [w463 w500 w526 w552]
        tunnel: w450 -> [_ _ _ _]
        tunnel: [w455 w494 w520 w546] -> w449
        tunnel: w448 -> [w462 w499 w525 w551]
        tunnel: [w461 w498 w524 w550] -> w447
        tunnel: w446 -> [w459 w496 w522 w548]
        tunnel: w445 -> [w457 w492 w519 w545]
        tunnel: [w456 w493 w518 w544] -> w444
        tunnel: w443 -> [w454 _ _ _]
        frame "ALL", Default {
          n82 = for {
            tunnel: w464 -> [w475]
            tunnel: w463 -> [w474]
            tunnel: w460 -> [w471]
            tunnel: w459 -> [w470] mode=indexing
            tunnel: w457 -> [w468]
            tunnel: [w467] -> w456
            tunnel: w462 -> [w473]
            tunnel: [w472] -> w461
            shift-right: [w466] -> w455
            shift-left: string[][] [] ("data") -> [w469]
            tunnel: w454 -> [w465]
            n83 = for {
              tunnel: w475 -> [w476]
              tunnel: w474 -> [w477]
              tunnel: w471 -> [_]
              tunnel: w470 -> [w489]
              shift-right: [w479] -> w466
              shift-left: w469 -> [w486]
              tunnel: w468 -> [w482]
              tunnel: [w481] -> w467
              tunnel: w473 -> [w484]
              tunnel: [w490] -> w472
              tunnel: w465 -> [w478] mode=indexing
              n84 = Concatenate Strings("Select DISTINCT PLAN_DATE,PRODUCTION_COUNT,STATION_ID,DATE from ", w489, " Where PLAN_DATE between '%s' and '%s' and STATION_ID = '%s' and SHIFT = '%s'") -> (w487:string)
              n85 = Format Into String(format string=w487, w477, w476, "2", w478) -> (resulting string=w491:string)  [unwired: 2 in, 1 out]
              n86 = call "Execute query.vi"("error in (no error)"=w482, "String"=w491, "connection reference"=w484) -> ("error out"=w481:errorcluster, "Table"=w485:string[][], "connection reference 2"=w490:T1)  [unwired: 3 in, 3 out]
              n87 = Build Array (concatenate)(w486, w485) -> (w479:string[][])
            }
          }
        }
        frame "1" {
          n88 = for {
            tunnel: w501 -> [w502]
            tunnel: w500 -> [w503]
            tunnel: w497 -> [w514]
            tunnel: w496 -> [w513] mode=indexing
            shift-right: [w515] -> w498
            shift-left: w499 -> [w517]
            shift-right: [w508] -> w494
            shift-left: string[][] [] ("data") -> [w510]
            tunnel: [w505] -> w493
            tunnel: w492 -> [w504]
            n89 = Concatenate Strings("Select DISTINCT PLAN_DATE,PRODUCTION_COUNT,STATION_ID,DATE from ", w513, " Where PLAN_DATE between '%s' and '%s' and SHIFT  ='%s' and STATION_ID ='%s'") -> (w511:string)
            n90 = Format Into String(format string=w511, w503, w502, w514, "2") -> (resulting string=w516:string)  [unwired: 2 in, 1 out]
            n91 = call "Execute query.vi"("error in (no error)"=w504, "String"=w516, "connection reference"=w517) -> ("error out"=w505:errorcluster, "Table"=w509:string[][], "connection reference 2"=w515:T1)  [unwired: 3 in, 3 out]
            n92 = Build Array (concatenate)(w510, w509) -> (w508:string[][])
          }
        }
        frame "2" {
          n93 = for {
            tunnel: w527 -> [w528]
            tunnel: w526 -> [w529]
            tunnel: w523 -> [w540]
            tunnel: w522 -> [w539] mode=indexing
            shift-right: [w541] -> w524
            shift-left: w525 -> [w543]
            shift-right: [w534] -> w520
            shift-left: string[][] [] ("data") -> [w536]
            tunnel: w519 -> [w531]
            tunnel: [w530] -> w518
            n94 = Concatenate Strings("Select DISTINCT PLAN_DATE,PRODUCTION_COUNT,STATION_ID,DATE from ", w539, " Where PLAN_DATE between '%s' and '%s' and SHIFT  ='%s' and STATION_ID ='%s'") -> (w537:string)
            n95 = Format Into String(format string=w537, w529, w528, w540, "2") -> (resulting string=w542:string)  [unwired: 2 in, 1 out]
            n96 = call "Execute query.vi"("error in (no error)"=w531, "String"=w542, "connection reference"=w543) -> ("error out"=w530:errorcluster, "Table"=w535:string[][], "connection reference 2"=w541:T1)  [unwired: 3 in, 3 out]
            n97 = Build Array (concatenate)(w536, w535) -> (w534:string[][])
          }
        }
        frame "3" {
          n98 = for {
            tunnel: w553 -> [w554]
            tunnel: w552 -> [w555]
            tunnel: w549 -> [w566]
            tunnel: w548 -> [w565] mode=indexing
            shift-right: [w567] -> w550
            shift-left: w551 -> [w569]
            shift-right: [w560] -> w546
            shift-left: string[][] [] ("data") -> [w562]
            tunnel: w545 -> [w557]
            tunnel: [w556] -> w544
            n99 = Concatenate Strings("Select DISTINCT PLAN_DATE,PRODUCTION_COUNT,STATION_ID,DATE from ", w565, " Where PLAN_DATE between '%s' and '%s' and SHIFT  ='%s' and STATION_ID ='%s'") -> (w563:string)
            n100 = Format Into String(format string=w563, w555, w554, w566, "2") -> (resulting string=w568:string)  [unwired: 2 in, 1 out]
            n101 = call "Execute query.vi"("error in (no error)"=w557, "String"=w568, "connection reference"=w569) -> ("error out"=w556:errorcluster, "Table"=w561:string[][], "connection reference 2"=w567:T1)  [unwired: 3 in, 3 out]
            n102 = Build Array (concatenate)(w562, w561) -> (w560:string[][])
          }
        }
      }
    }
    frame "ST 3" {
      n103 = case shown="\"ALL\", Default" w580 {
        selector: w580 -> [w587 w624 w650 w676]
        tunnel: w579 -> [w591 w628 w654 w680]
        tunnel: w578 -> [w590 w627 w653 w679]
        tunnel: w577 -> [_ _ _ _]
        tunnel: [w582 w621 w647 w673] -> w576
        tunnel: w575 -> [w589 w626 w652 w678]
        tunnel: [w588 w625 w651 w677] -> w574
        tunnel: w573 -> [w586 w623 w649 w675]
        tunnel: w572 -> [w584 w619 w646 w672]
        tunnel: [w583 w620 w645 w671] -> w571
        tunnel: w570 -> [w581 _ _ _]
        frame "ALL", Default {
          n104 = for {
            tunnel: w591 -> [w602]
            tunnel: w590 -> [w601]
            tunnel: w587 -> [w598]
            tunnel: w586 -> [w597] mode=indexing
            tunnel: w584 -> [w595]
            tunnel: [w594] -> w583
            tunnel: w589 -> [w600]
            tunnel: [w599] -> w588
            shift-right: [w593] -> w582
            shift-left: string[][] [] ("data") -> [w596]
            tunnel: w581 -> [w592]
            n105 = for {
              tunnel: w602 -> [w603]
              tunnel: w601 -> [w604]
              tunnel: w598 -> [_]
              tunnel: w597 -> [w616]
              shift-right: [w606] -> w593
              shift-left: w596 -> [w613]
              tunnel: w595 -> [w609]
              tunnel: [w608] -> w594
              tunnel: w600 -> [w611]
              tunnel: [w617] -> w599
              tunnel: w592 -> [w605] mode=indexing
              n106 = Concatenate Strings("Select DISTINCT PLAN_DATE,PRODUCTION_COUNT,STATION_ID,DATE from ", w616, " Where PLAN_DATE between '%s' and '%s' and STATION_ID = '%s' and SHIFT = '%s'") -> (w614:string)
              n107 = Format Into String(format string=w614, w604, w603, "3", w605) -> (resulting string=w618:string)  [unwired: 2 in, 1 out]
              n108 = call "Execute query.vi"("error in (no error)"=w609, "String"=w618, "connection reference"=w611) -> ("error out"=w608:errorcluster, "Table"=w612:string[][], "connection reference 2"=w617:T1)  [unwired: 3 in, 3 out]
              n109 = Build Array (concatenate)(w613, w612) -> (w606:string[][])
            }
          }
        }
        frame "1" {
          n110 = for {
            tunnel: w628 -> [w629]
            tunnel: w627 -> [w630]
            tunnel: w624 -> [w641]
            tunnel: w623 -> [w640] mode=indexing
            shift-right: [w642] -> w625
            shift-left: w626 -> [w644]
            shift-right: [w635] -> w621
            shift-left: string[][] [] ("data") -> [w637]
            tunnel: [w632] -> w620
            tunnel: w619 -> [w631]
            n111 = Concatenate Strings("Select DISTINCT PLAN_DATE,PRODUCTION_COUNT,STATION_ID,DATE from ", w640, " Where PLAN_DATE between '%s' and '%s' and SHIFT  ='%s' and STATION_ID ='%s'") -> (w638:string)
            n112 = Format Into String(format string=w638, w630, w629, w641, "3") -> (resulting string=w643:string)  [unwired: 2 in, 1 out]
            n113 = call "Execute query.vi"("error in (no error)"=w631, "String"=w643, "connection reference"=w644) -> ("error out"=w632:errorcluster, "Table"=w636:string[][], "connection reference 2"=w642:T1)  [unwired: 3 in, 3 out]
            n114 = Build Array (concatenate)(w637, w636) -> (w635:string[][])
          }
        }
        frame "2" {
          n115 = for {
            tunnel: w654 -> [w655]
            tunnel: w653 -> [w656]
            tunnel: w650 -> [w667]
            tunnel: w649 -> [w666] mode=indexing
            shift-right: [w668] -> w651
            shift-left: w652 -> [w670]
            shift-right: [w661] -> w647
            shift-left: string[][] [] ("data") -> [w663]
            tunnel: w646 -> [w658]
            tunnel: [w657] -> w645
            n116 = Concatenate Strings("Select DISTINCT PLAN_DATE,PRODUCTION_COUNT,STATION_ID,DATE from ", w666, " Where PLAN_DATE between '%s' and '%s' and SHIFT  ='%s' and STATION_ID ='%s'") -> (w664:string)
            n117 = Format Into String(format string=w664, w656, w655, w667, "3") -> (resulting string=w669:string)  [unwired: 2 in, 1 out]
            n118 = call "Execute query.vi"("error in (no error)"=w658, "String"=w669, "connection reference"=w670) -> ("error out"=w657:errorcluster, "Table"=w662:string[][], "connection reference 2"=w668:T1)  [unwired: 3 in, 3 out]
            n119 = Build Array (concatenate)(w663, w662) -> (w661:string[][])
          }
        }
        frame "3" {
          n120 = for {
            tunnel: w680 -> [w681]
            tunnel: w679 -> [w682]
            tunnel: w676 -> [w693]
            tunnel: w675 -> [w692] mode=indexing
            shift-right: [w694] -> w677
            shift-left: w678 -> [w696]
            shift-right: [w687] -> w673
            shift-left: string[][] [] ("data") -> [w689]
            tunnel: w672 -> [w684]
            tunnel: [w683] -> w671
            n121 = Concatenate Strings("Select DISTINCT PLAN_DATE,PRODUCTION_COUNT,STATION_ID,DATE from ", w692, " Where PLAN_DATE between '%s' and '%s' and SHIFT  ='%s' and STATION_ID ='%s'") -> (w690:string)
            n122 = Format Into String(format string=w690, w682, w681, w693, "3") -> (resulting string=w695:string)  [unwired: 2 in, 1 out]
            n123 = call "Execute query.vi"("error in (no error)"=w684, "String"=w695, "connection reference"=w696) -> ("error out"=w683:errorcluster, "Table"=w688:string[][], "connection reference 2"=w694:T1)  [unwired: 3 in, 3 out]
            n124 = Build Array (concatenate)(w689, w688) -> (w687:string[][])
          }
        }
      }
    }
    frame "ST 4" {
      (unwired) "Select DISTINCT PLAN_DATE,PRODUCTION_COUNT,STATION_ID,SHIFT,DATE from "
      (unwired) " Where PLAN_DATE between '%s' and '%s' and STATION_ID = '%d' and SHIFT = '%d'"
      n125 = case shown="\"1\"" w707 {
        selector: w707 -> [w714 w751 w777 w803]
        tunnel: w706 -> [w718 w755 w781 w807]
        tunnel: w705 -> [w717 w754 w780 w806]
        tunnel: w704 -> [_ _ _ _]
        tunnel: [w709 w748 w774 w800] -> w703
        tunnel: w702 -> [w716 w753 w779 w805]
        tunnel: [w715 w752 w778 w804] -> w701
        tunnel: w700 -> [w713 w750 w776 w802]
        tunnel: w699 -> [w711 w746 w773 w799]
        tunnel: [w710 w747 w772 w798] -> w698
        tunnel: w697 -> [w708 _ _ _]
        frame "ALL", Default {
          n126 = for {
            tunnel: w718 -> [w729]
            tunnel: w717 -> [w728]
            tunnel: w714 -> [w725]
            tunnel: w713 -> [w724] mode=indexing
            tunnel: w711 -> [w722]
            tunnel: [w721] -> w710
            tunnel: w716 -> [w727]
            tunnel: [w726] -> w715
            shift-right: [w720] -> w709
            shift-left: string[][] [] ("data") -> [w723]
            tunnel: w708 -> [w719]
            n127 = for {
              tunnel: w729 -> [w730]
              tunnel: w728 -> [w731]
              tunnel: w725 -> [_]
              tunnel: w724 -> [w743]
              shift-right: [w733] -> w720
              shift-left: w723 -> [w740]
              tunnel: w722 -> [w736]
              tunnel: [w735] -> w721
              tunnel: w727 -> [w738]
              tunnel: [w744] -> w726
              tunnel: w719 -> [w732] mode=indexing
              n128 = Concatenate Strings("Select DISTINCT PLAN_DATE,PRODUCTION_COUNT,STATION_ID,DATE from ", w743, " Where PLAN_DATE between '%s' and '%s' and STATION_ID = '%s' and SHIFT = '%s'") -> (w741:string)
              n129 = Format Into String(format string=w741, w731, w730, "4", w732) -> (resulting string=w745:string)  [unwired: 2 in, 1 out]
              n130 = call "Execute query.vi"("error in (no error)"=w736, "String"=w745, "connection reference"=w738) -> ("error out"=w735:errorcluster, "Table"=w739:string[][], "connection reference 2"=w744:T1)  [unwired: 3 in, 3 out]
              n131 = Build Array (concatenate)(w740, w739) -> (w733:string[][])
            }
          }
        }
        frame "1" {
          n132 = for {
            tunnel: w755 -> [w756]
            tunnel: w754 -> [w757]
            tunnel: w751 -> [w768]
            tunnel: w750 -> [w767] mode=indexing
            shift-right: [w769] -> w752
            shift-left: w753 -> [w771]
            shift-right: [w762] -> w748
            shift-left: string[][] [] ("data") -> [w764]
            tunnel: [w759] -> w747
            tunnel: w746 -> [w758]
            n133 = Concatenate Strings("Select DISTINCT PLAN_DATE,PRODUCTION_COUNT,STATION_ID,DATE from ", w767, " Where PLAN_DATE between '%s' and '%s' and SHIFT  ='%s' and STATION_ID ='%s'") -> (w765:string)
            n134 = Format Into String(format string=w765, w757, w756, w768, "4") -> (resulting string=w770:string)  [unwired: 2 in, 1 out]
            n135 = call "Execute query.vi"("error in (no error)"=w758, "String"=w770, "connection reference"=w771) -> ("error out"=w759:errorcluster, "Table"=w763:string[][], "connection reference 2"=w769:T1)  [unwired: 3 in, 3 out]
            n136 = Build Array (concatenate)(w764, w763) -> (w762:string[][])
          }
        }
        frame "2" {
          n137 = for {
            tunnel: w781 -> [w782]
            tunnel: w780 -> [w783]
            tunnel: w777 -> [w794]
            tunnel: w776 -> [w793] mode=indexing
            shift-right: [w795] -> w778
            shift-left: w779 -> [w797]
            shift-right: [w788] -> w774
            shift-left: string[][] [] ("data") -> [w790]
            tunnel: w773 -> [w785]
            tunnel: [w784] -> w772
            n138 = Concatenate Strings("Select DISTINCT PLAN_DATE,PRODUCTION_COUNT,STATION_ID,DATE from ", w793, " Where PLAN_DATE between '%s' and '%s' and SHIFT  ='%s' and STATION_ID ='%s'") -> (w791:string)
            n139 = Format Into String(format string=w791, w783, w782, w794, "4") -> (resulting string=w796:string)  [unwired: 2 in, 1 out]
            n140 = call "Execute query.vi"("error in (no error)"=w785, "String"=w796, "connection reference"=w797) -> ("error out"=w784:errorcluster, "Table"=w789:string[][], "connection reference 2"=w795:T1)  [unwired: 3 in, 3 out]
            n141 = Build Array (concatenate)(w790, w789) -> (w788:string[][])
          }
        }
        frame "3" {
          n142 = for {
            tunnel: w807 -> [w808]
            tunnel: w806 -> [w809]
            tunnel: w803 -> [w820]
            tunnel: w802 -> [w819] mode=indexing
            shift-right: [w821] -> w804
            shift-left: w805 -> [w823]
            shift-right: [w814] -> w800
            shift-left: string[][] [] ("data") -> [w816]
            tunnel: w799 -> [w811]
            tunnel: [w810] -> w798
            n143 = Concatenate Strings("Select DISTINCT PLAN_DATE,PRODUCTION_COUNT,STATION_ID,DATE from ", w819, " Where PLAN_DATE between '%s' and '%s' and SHIFT  ='%s' and STATION_ID ='%s'") -> (w817:string)
            n144 = Format Into String(format string=w817, w809, w808, w820, "4") -> (resulting string=w822:string)  [unwired: 2 in, 1 out]
            n145 = call "Execute query.vi"("error in (no error)"=w811, "String"=w822, "connection reference"=w823) -> ("error out"=w810:errorcluster, "Table"=w815:string[][], "connection reference 2"=w821:T1)  [unwired: 3 in, 3 out]
            n146 = Build Array (concatenate)(w816, w815) -> (w814:string[][])
          }
        }
      }
    }
    frame "ST 5" {
      (unwired) "Select DISTINCT PLAN_DATE,PRODUCTION_COUNT,STATION_ID,SHIFT,DATE from "
      (unwired) " Where PLAN_DATE between '%s' and '%s' and STATION_ID = '%d' and SHIFT = '%d'"
      n147 = case shown="\"ALL\", Default" w834 {
        selector: w834 -> [w841 w878 w904 w930]
        tunnel: w833 -> [w845 w882 w908 w934]
        tunnel: w832 -> [w844 w881 w907 w933]
        tunnel: w831 -> [_ _ _ _]
        tunnel: [w836 w875 w901 w927] -> w830
        tunnel: w829 -> [w843 w880 w906 w932]
        tunnel: [w842 w879 w905 w931] -> w828
        tunnel: w827 -> [w840 w877 w903 w929]
        tunnel: w826 -> [w838 w873 w900 w926]
        tunnel: [w837 w874 w899 w925] -> w825
        tunnel: w824 -> [w835 _ _ _]
        frame "ALL", Default {
          n148 = for {
            tunnel: w845 -> [w856]
            tunnel: w844 -> [w855]
            tunnel: w841 -> [w852]
            tunnel: w840 -> [w851] mode=indexing
            tunnel: w838 -> [w849]
            tunnel: [w848] -> w837
            tunnel: w843 -> [w854]
            tunnel: [w853] -> w842
            shift-right: [w847] -> w836
            shift-left: string[][] [] ("data") -> [w850]
            tunnel: w835 -> [w846]
            n149 = for {
              tunnel: w856 -> [w857]
              tunnel: w855 -> [w858]
              tunnel: w852 -> [_]
              tunnel: w851 -> [w870]
              shift-right: [w860] -> w847
              shift-left: w850 -> [w867]
              tunnel: w849 -> [w863]
              tunnel: [w862] -> w848
              tunnel: w854 -> [w865]
              tunnel: [w871] -> w853
              tunnel: w846 -> [w859] mode=indexing
              n150 = Concatenate Strings("Select DISTINCT PLAN_DATE,PRODUCTION_COUNT,STATION_ID,DATE from ", w870, " Where PLAN_DATE between '%s' and '%s' and STATION_ID = '%s' and SHIFT = '%s'") -> (w868:string)
              n151 = Format Into String(format string=w868, w858, w857, "5", w859) -> (resulting string=w872:string)  [unwired: 2 in, 1 out]
              n152 = call "Execute query.vi"("error in (no error)"=w863, "String"=w872, "connection reference"=w865) -> ("error out"=w862:errorcluster, "Table"=w866:string[][], "connection reference 2"=w871:T1)  [unwired: 3 in, 3 out]
              n153 = Build Array (concatenate)(w867, w866) -> (w860:string[][])
            }
          }
        }
        frame "1" {
          n154 = for {
            tunnel: w882 -> [w883]
            tunnel: w881 -> [w884]
            tunnel: w878 -> [w895]
            tunnel: w877 -> [w894] mode=indexing
            shift-right: [w896] -> w879
            shift-left: w880 -> [w898]
            shift-right: [w889] -> w875
            shift-left: string[][] [] ("data") -> [w891]
            tunnel: [w886] -> w874
            tunnel: w873 -> [w885]
            n155 = Concatenate Strings("Select DISTINCT PLAN_DATE,PRODUCTION_COUNT,STATION_ID,DATE from ", w894, " Where PLAN_DATE between '%s' and '%s' and SHIFT  ='%s' and STATION_ID ='%s'") -> (w892:string)
            n156 = Format Into String(format string=w892, w884, w883, w895, "5") -> (resulting string=w897:string)  [unwired: 2 in, 1 out]
            n157 = call "Execute query.vi"("error in (no error)"=w885, "String"=w897, "connection reference"=w898) -> ("error out"=w886:errorcluster, "Table"=w890:string[][], "connection reference 2"=w896:T1)  [unwired: 3 in, 3 out]
            n158 = Build Array (concatenate)(w891, w890) -> (w889:string[][])
          }
        }
        frame "2" {
          n159 = for {
            tunnel: w908 -> [w909]
            tunnel: w907 -> [w910]
            tunnel: w904 -> [w921]
            tunnel: w903 -> [w920] mode=indexing
            shift-right: [w922] -> w905
            shift-left: w906 -> [w924]
            shift-right: [w915] -> w901
            shift-left: string[][] [] ("data") -> [w917]
            tunnel: w900 -> [w912]
            tunnel: [w911] -> w899
            n160 = Concatenate Strings("Select DISTINCT PLAN_DATE,PRODUCTION_COUNT,STATION_ID,DATE from ", w920, " Where PLAN_DATE between '%s' and '%s' and SHIFT  ='%s' and STATION_ID ='%s'") -> (w918:string)
            n161 = Format Into String(format string=w918, w910, w909, w921, "5") -> (resulting string=w923:string)  [unwired: 2 in, 1 out]
            n162 = call "Execute query.vi"("error in (no error)"=w912, "String"=w923, "connection reference"=w924) -> ("error out"=w911:errorcluster, "Table"=w916:string[][], "connection reference 2"=w922:T1)  [unwired: 3 in, 3 out]
            n163 = Build Array (concatenate)(w917, w916) -> (w915:string[][])
          }
        }
        frame "3" {
          n164 = for {
            tunnel: w934 -> [w935]
            tunnel: w933 -> [w936]
            tunnel: w930 -> [w947]
            tunnel: w929 -> [w946] mode=indexing
            shift-right: [w948] -> w931
            shift-left: w932 -> [w950]
            shift-right: [w941] -> w927
            shift-left: string[][] [] ("data") -> [w943]
            tunnel: w926 -> [w938]
            tunnel: [w937] -> w925
            n165 = Concatenate Strings("Select DISTINCT PLAN_DATE,PRODUCTION_COUNT,STATION_ID,DATE from ", w946, " Where PLAN_DATE between '%s' and '%s' and SHIFT  ='%s' and STATION_ID ='%s'") -> (w944:string)
            n166 = Format Into String(format string=w944, w936, w935, w947, "5") -> (resulting string=w949:string)  [unwired: 2 in, 1 out]
            n167 = call "Execute query.vi"("error in (no error)"=w938, "String"=w949, "connection reference"=w950) -> ("error out"=w937:errorcluster, "Table"=w942:string[][], "connection reference 2"=w948:T1)  [unwired: 3 in, 3 out]
            n168 = Build Array (concatenate)(w943, w942) -> (w941:string[][])
          }
        }
      }
    }
    frame "ST 6" {
      (unwired) "Select DISTINCT PLAN_DATE,PRODUCTION_COUNT,STATION_ID,SHIFT,DATE from "
      (unwired) " Where PLAN_DATE between '%s' and '%s' and STATION_ID = '%d' and SHIFT = '%d'"
      n169 = case shown="\"ALL\", Default" w961 {
        selector: w961 -> [w968 w1005 w1031 w1057]
        tunnel: w960 -> [w972 w1009 w1035 w1061]
        tunnel: w959 -> [w971 w1008 w1034 w1060]
        tunnel: w958 -> [_ _ _ _]
        tunnel: [w963 w1002 w1028 w1054] -> w957
        tunnel: w956 -> [w970 w1007 w1033 w1059]
        tunnel: [w969 w1006 w1032 w1058] -> w955
        tunnel: w954 -> [w967 w1004 w1030 w1056]
        tunnel: w953 -> [w965 w1000 w1027 w1053]
        tunnel: [w964 w1001 w1026 w1052] -> w952
        tunnel: w951 -> [w962 _ _ _]
        frame "ALL", Default {
          n170 = for {
            tunnel: w972 -> [w983]
            tunnel: w971 -> [w982]
            tunnel: w968 -> [w979]
            tunnel: w967 -> [w978] mode=indexing
            tunnel: w965 -> [w976]
            tunnel: [w975] -> w964
            tunnel: w970 -> [w981]
            tunnel: [w980] -> w969
            shift-right: [w974] -> w963
            shift-left: string[][] [] ("data") -> [w977]
            tunnel: w962 -> [w973]
            n171 = for {
              tunnel: w983 -> [w984]
              tunnel: w982 -> [w985]
              tunnel: w979 -> [_]
              tunnel: w978 -> [w997]
              shift-right: [w987] -> w974
              shift-left: w977 -> [w994]
              tunnel: w976 -> [w990]
              tunnel: [w989] -> w975
              tunnel: w981 -> [w992]
              tunnel: [w998] -> w980
              tunnel: w973 -> [w986] mode=indexing
              n172 = Concatenate Strings("Select DISTINCT PLAN_DATE,PRODUCTION_COUNT,STATION_ID,DATE from ", w997, " Where PLAN_DATE between '%s' and '%s' and STATION_ID = '%s' and SHIFT = '%s'") -> (w995:string)
              n173 = Format Into String(format string=w995, w985, w984, "6", w986) -> (resulting string=w999:string)  [unwired: 2 in, 1 out]
              n174 = call "Execute query.vi"("error in (no error)"=w990, "String"=w999, "connection reference"=w992) -> ("error out"=w989:errorcluster, "Table"=w993:string[][], "connection reference 2"=w998:T1)  [unwired: 3 in, 3 out]
              n175 = Build Array (concatenate)(w994, w993) -> (w987:string[][])
            }
          }
        }
        frame "1" {
          n176 = for {
            tunnel: w1009 -> [w1010]
            tunnel: w1008 -> [w1011]
            tunnel: w1005 -> [w1022]
            tunnel: w1004 -> [w1021] mode=indexing
            shift-right: [w1023] -> w1006
            shift-left: w1007 -> [w1025]
            shift-right: [w1016] -> w1002
            shift-left: string[][] [] ("data") -> [w1018]
            tunnel: [w1013] -> w1001
            tunnel: w1000 -> [w1012]
            n177 = Concatenate Strings("Select DISTINCT PLAN_DATE,PRODUCTION_COUNT,STATION_ID,DATE from ", w1021, " Where PLAN_DATE between '%s' and '%s' and SHIFT  ='%s' and STATION_ID ='%s'") -> (w1019:string)
            n178 = Format Into String(format string=w1019, w1011, w1010, w1022, "6") -> (resulting string=w1024:string)  [unwired: 2 in, 1 out]
            n179 = call "Execute query.vi"("error in (no error)"=w1012, "String"=w1024, "connection reference"=w1025) -> ("error out"=w1013:errorcluster, "Table"=w1017:string[][], "connection reference 2"=w1023:T1)  [unwired: 3 in, 3 out]
            n180 = Build Array (concatenate)(w1018, w1017) -> (w1016:string[][])
          }
        }
        frame "2" {
          n181 = for {
            tunnel: w1035 -> [w1036]
            tunnel: w1034 -> [w1037]
            tunnel: w1031 -> [w1048]
            tunnel: w1030 -> [w1047] mode=indexing
            shift-right: [w1049] -> w1032
            shift-left: w1033 -> [w1051]
            shift-right: [w1042] -> w1028
            shift-left: string[][] [] ("data") -> [w1044]
            tunnel: w1027 -> [w1039]
            tunnel: [w1038] -> w1026
            n182 = Concatenate Strings("Select DISTINCT PLAN_DATE,PRODUCTION_COUNT,STATION_ID,DATE from ", w1047, " Where PLAN_DATE between '%s' and '%s' and SHIFT  ='%s' and STATION_ID ='%s'") -> (w1045:string)
            n183 = Format Into String(format string=w1045, w1037, w1036, w1048, "6") -> (resulting string=w1050:string)  [unwired: 2 in, 1 out]
            n184 = call "Execute query.vi"("error in (no error)"=w1039, "String"=w1050, "connection reference"=w1051) -> ("error out"=w1038:errorcluster, "Table"=w1043:string[][], "connection reference 2"=w1049:T1)  [unwired: 3 in, 3 out]
            n185 = Build Array (concatenate)(w1044, w1043) -> (w1042:string[][])
          }
        }
        frame "3" {
          n186 = for {
            tunnel: w1061 -> [w1062]
            tunnel: w1060 -> [w1063]
            tunnel: w1057 -> [w1074]
            tunnel: w1056 -> [w1073] mode=indexing
            shift-right: [w1075] -> w1058
            shift-left: w1059 -> [w1077]
            shift-right: [w1068] -> w1054
            shift-left: string[][] [] ("data") -> [w1070]
            tunnel: w1053 -> [w1065]
            tunnel: [w1064] -> w1052
            n187 = Concatenate Strings("Select DISTINCT PLAN_DATE,PRODUCTION_COUNT,STATION_ID,DATE from ", w1073, " Where PLAN_DATE between '%s' and '%s' and SHIFT  ='%s' and STATION_ID ='%s'") -> (w1071:string)
            n188 = Format Into String(format string=w1071, w1063, w1062, w1074, "6") -> (resulting string=w1076:string)  [unwired: 2 in, 1 out]
            n189 = call "Execute query.vi"("error in (no error)"=w1065, "String"=w1076, "connection reference"=w1077) -> ("error out"=w1064:errorcluster, "Table"=w1069:string[][], "connection reference 2"=w1075:T1)  [unwired: 3 in, 3 out]
            n190 = Build Array (concatenate)(w1070, w1069) -> (w1068:string[][])
          }
        }
      }
    }
  }
  "Table" <- w18
  "Refnum out" <- w47
  "ALL IN ONE" <- w36
  n191 = Merge Errors(w29, w28) -> (→"error out":errorcluster)
  n192 = Index Array(array=w18, index (col)=0 ("disabled index (col)")) -> (element=w9:string[])  [unwired: 1 in]
  n193 = call "Search_1d_array_element.vi"("Count in"=string[] [] ("Count"), "BD Date"=w9, "Elements Found in"=string[] [] ("Elements Found")) -> ("Elements Found out"=w2:string[])  [unwired: 4 in, 2 out]
  "Elements Found out" <- w2
  n194 = Fract/Exp String To Number(string=w18) -> (number=w17:dbl[][])  [unwired: 3 in, 1 out]
  n195 = Array Size(array=w17) -> (size(s)=w25:i32[])
  n196 = Index Array(array=w25) -> (element #1=w23:i32, element #2=w19:i32)  [unwired: 2 in]
  n197 = Initialize Array(0.0, w23, w19) -> (w24:dbl[][])
  n198 = for {
    N: w23 -> [_]
    shift-right: [w1084] -> w20
    shift-left: w24 -> [w1083]
    shift-right: [w1081] -> w21
    shift-left: 0 -> [w1082]
    tunnel: w17 -> [w1079] mode=indexing
    n199 = Not Equal To 0?(x=w1079) -> (x != 0?=w1080:bool[])
    n200 = And Array Elements(Boolean array=w1080) -> (logical AND=w1078:bool)
    n201 = case shown="True" w1078 {
      tunnel: w1083 -> [w1086 w1091]
      tunnel: [w1086 w1090] -> w1084
      tunnel: w1082 -> [w1085 w1088]
      tunnel: [w1085 w1089] -> w1081
      tunnel: w1079 -> [_ w1087]
      frame False {
      }
      frame True {
        n202 = Increment(x=w1088) -> (x+1=w1089:i32)
        n203 = Replace Array Subset(array=w1091, new element=w1087, index (row)=w1088) -> (w1090:dbl[][])  [unwired: 1 in]
      }
    }
  }
  n204 = Reshape Array(w20, w21, w19) -> (w14:dbl[][])
  n205 = Number To Fractional String(number=w14, precision (6)=i16 0) -> (F-format string=w13:string[][])  [unwired: 2 in]
  n206 = Index Array(array=w13, index (col)=3 ("disabled index (col)")) -> (element=w12:string[])  [unwired: 1 in]
  n207 = call "Search_1d_array_element.vi"("Count in"=string[] [] ("Count"), "BD Date"=w12, "Elements Found in"=string[] [] ("Elements Found")) -> ("Count out"=w39:string[])  [unwired: 4 in, 2 out]
  "PROD_COUNT TEST" <- w39
  n208 = disable-structure shown="Enabled" {
    disable-tunnel: [w1096 _] -> w42
    disable-tunnel: w39 -> [w1095 _]
    disable-tunnel: [w1094 _] -> w38
    disable-tunnel: w18 -> [w1093 w1099]
    disable-tunnel: w2 -> [w1092 _]
    disable-tunnel: [_ w1097] -> w1
    frame Disabled {
      n209 = call "Production_count_sum.vi"("PROD_COUNT"=w1095, "Table 3"=w1093, "date count"=w1095, "Founded dates"=w1092) -> ("sum"=w1096:i32[], "Array 3"=w1094:string[][])  [unwired: 6 in]
    }
    frame Enabled {
      n210 = Array Size(array=w1099) -> (size(s)=w1098:i32[])
      n211 = Index Array(array=w1098) -> (element #1=w1097:i32)  [unwired: 2 in, 1 out]
    }
  }
  "sum" <- w42
  "Array 3" <- w38
  "Count" <- w1
